vi "main（新）线程二.vi"(8 "停止 2":bool, 11 "线程选择":string(combo)) -> ()   [LabVIEW 2016]
uses:
  <vilib>/Averna/Notify Icon/NotifyIcon.llb/BalloonIcon.ctl
  <vilib>/Utility/miscctls.llb/LVPointTypeDef.ctl
  <vilib>/Utility/config.llb/Read Key (String).vi
  <vilib>/Utility/config.llb/Read Key (I32).vi
  <vilib>/Utility/config.llb/Write Key (String).vi
  <vilib>/Utility/config.llb/Write Key (U32).vi
  <vilib>/Averna/Notify Icon/NotifyIcon.llb/GetSelectedItemEvent.vi
  <vilib>/Averna/Notify Icon/NotifyIcon.llb/SetVisible.vi
  <vilib>/Averna/Notify Icon/NotifyIcon.llb/SetMenuDefaultItem.vi
  <vilib>/Averna/Notify Icon/NotifyIcon.llb/SetTipText.vi
  <vilib>/Averna/Notify Icon/NotifyIcon.llb/NotifyIcon.lvclass
  <vilib>/Utility/config.llb/NI_LVConfig.lvlib
  data/FreeMem.dll
  <vilib>/ptbypt/NI_PtbyPt.lvlib
panel:
  in  "系统编码选择框":string(combo)="地表水质量监测"
  out "主队列输出":refnum<queue>
  out "软件版本":string
  out "数据接收中断 2":bool=TRUE
  out "掉线指示":bool
  out "数据上传":bool
  out "通信状态":bool
  in  "TCP掉线时间节点":string
  out "TCP服务端掉线计数":i32
  out "元素":string
  out "步骤":T1(ring)
  out "1st Error to Convert":i32(ring)=56 items=["无错误", "参数错误", "内存已满", "超出区域", "文件结束", "文件已打开", "一般文件IO错误", "未找到文件", "文件权限错误", "磁盘已满", "路径副本", "打开过多文件", "未启用", "未找到资源文件", "无法添加资源", "未找到资源", "未找到图像", "图像内存错误", "画笔不存在", "配置错误类型", "配置未找到解析段", "配置解析错误", "配置内存错误", "错误外部代码格式", "错误外部代码偏移量", "外部代码不存在", "空窗口", "销毁窗口错误", "空菜单", "打印已中止", "错误打印记录", "打印驱动程序错误", "打印时窗口错误", "打印时内存错误", "打印对话框错误", "一般打印错误", "无效设备引用句柄", "设备未找到", "设备参数错误", "设备单位错误", "无法打开设备", "设备调用已中止", "一般错误", "用户已取消", "对象ID过低", "对象ID过高", "对象不在堆中", "未知的堆", "错误DefProc ID", "DefProc不在表格中", "范围外信息", "空方法", "未知信息", "不支持管理器调用", "错误地址", "连接过程中", "连接超时", "连接过程中", "不支持网络属性", "网络错误", "正在使用的地址", "系统缺少内存", "连接已中止", "连接已拒绝", "连接未建立", "连接已建立", "连接已关闭", "初始化错误（交互应用程序管理器）", "错误事件发生", "等待无约束事件发生处理程序", "事件发生队列溢出", "错误路径", "未发出信号量", "未识别类型（交互应用程序管理器）"]
  out "重发数据":bool
  in  "确定":bool
  out "配置信息":T2
  in  "返回":bool
  in  "参数配置":bool
  in  "PW1":string
  in  "MN1":string
  in  "PORT1":string
  in  "IP1":string
  in  "站点设备1":string
  in  "站点名称1":string
  in  "站点设备":string(combo)="古田污水厂5号"
  in  "站点名称":string(combo)="古田"
  in  "port":string(combo)="1000"
  in  "IP":string(combo)="127.0.0.1"
  in  "PW":string
  in  "MN":string
  out "设置超时时间/min":i32=1
  in  "实时数据发送时间间隔/min":u32=10
  in  "配置模式":u16(ring) items=["现有参数", "自主输入"]
  out "连接的字符串":string
  out "参数":string
  out "data":string[][](table)
  out "数据发送重叠":bool
  out "数据接收中断":bool=TRUE
  out "数据正在发送":bool=TRUE
  out "QN":string
  out "时间QN":string
  out "系统编码ST":string
  out "命令编码CN":string
  out "密码PW":string
  out "设备编码MN":string
  out "拆分包及应答Flag":string
  out "数据":string
  in  "实时数据参数选择框":T3={"水样测量数据"=TRUE, "零点核查数据"=TRUE, "跨度核查数据"=TRUE, "加标回收数据"=TRUE, "平行样数据"=FALSE}
  out "运行时间次数":i32
  out "数据输出":string
  out "try":dbl
  in  "table元素":string
  out "读取报文显示":string
  out "发送报文显示":string
  out "数组":string[](array[string])
  out "数组 2":string[](array[string])
  out "空闲时间":dbl
  out "心跳包":bool
  out "时间标识":timestamp format="%<%Y/%m/%d %H:%M:%S>T"
  in  "连接ID":refnum<k5>
  out "错误输出":errorcluster
  out "主动上传数据次数":i32
  out "error out":errorcluster
  # "192.168.165.122"
  # "3300"
  # "已经实现的功能：发送实时数据、读取小时数据、反控指令、读取核查数据"
  # "数据发送间隔时间必须要小于数采仪出数据的时间间隔"
  # "读取发送的参数要可选择，包括：参数名、因子编码"
  # "参数配置"
  # "站点名称"
  # "站点设备"
  # "IP"
  # "PORT"
  # "MN"
  # "PW"
  # "读取的参数区"
  # "水样测量数据"
  # "零点核查数据"
  # "跨度核查数据"
  # "加标回收数据"
  # "平行样数据"
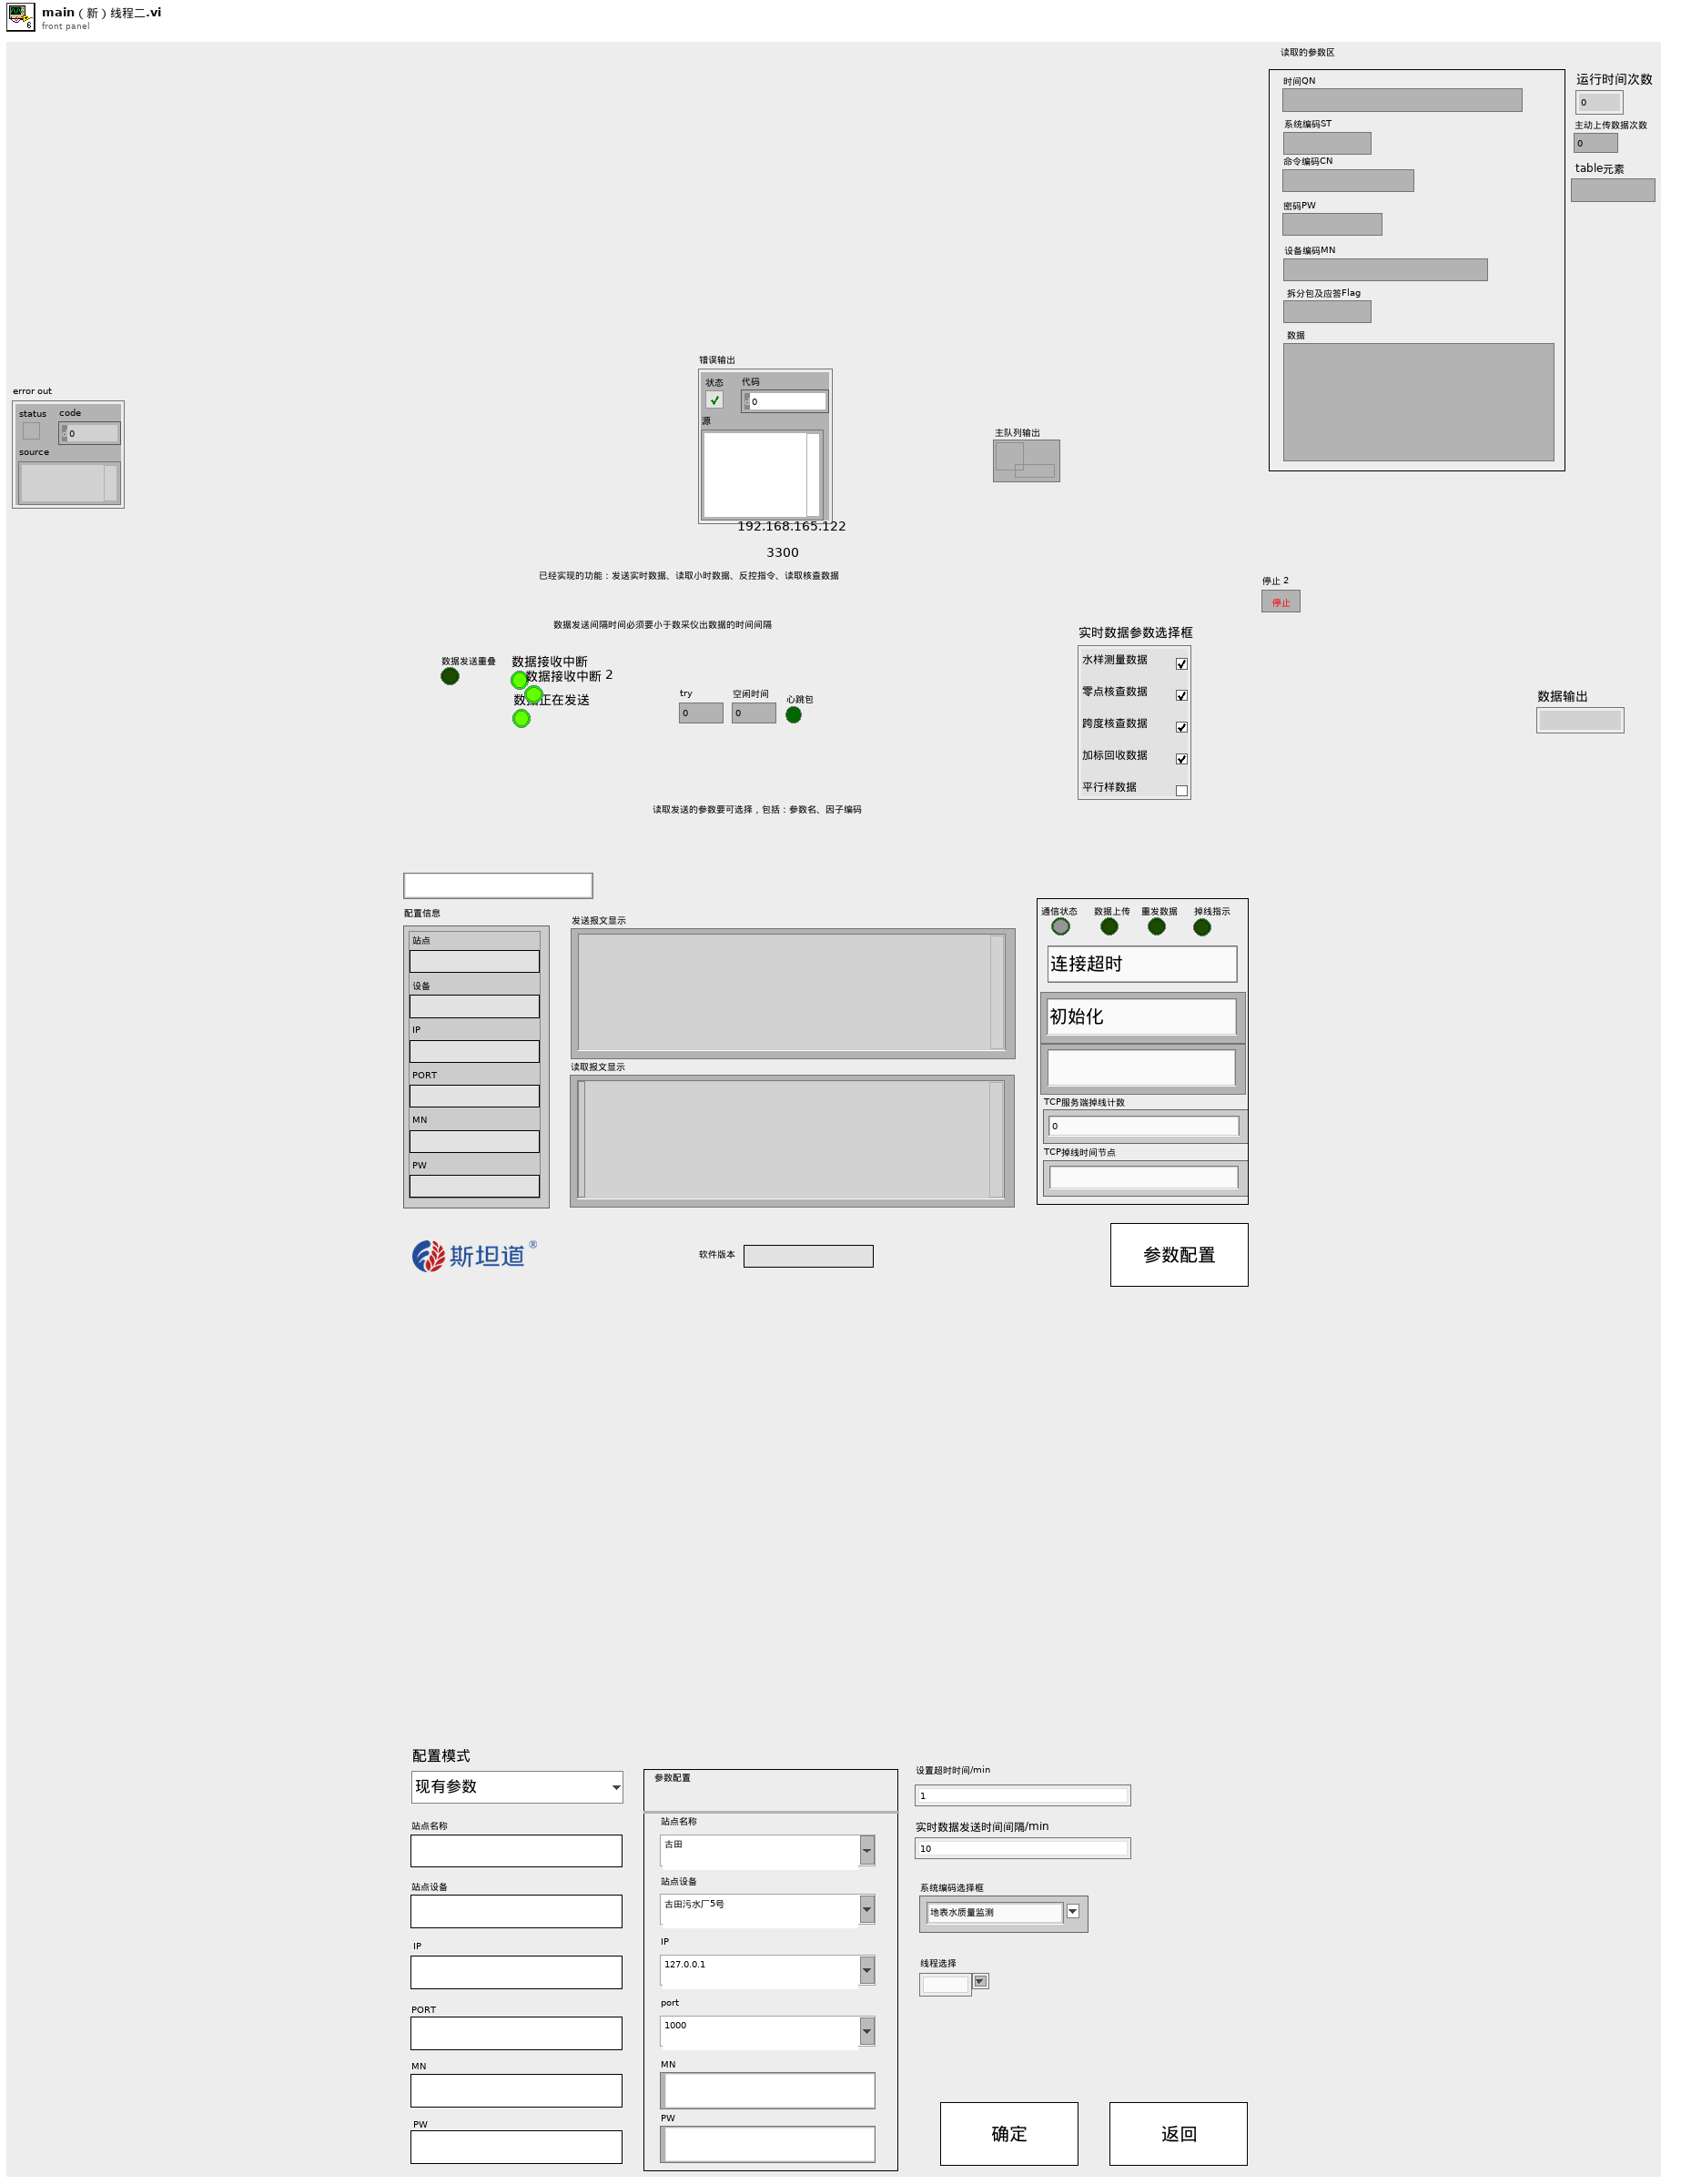
[diagram p1: front panel]
types:
  T1 = enum16{"初始化", "打开连接", "表格比对", "发送数据", "读取数据", "数据处理"}
  T2 = cluster{"站点":string, "设备":string, "IP":string, "PORT":string, "MN":string, "PW":string}
  T3 = cluster{"水样测量数据":bool, "零点核查数据":bool, "跨度核查数据":bool, "加标回收数据":bool, "平行样数据":bool}
  T4 = enum32{"Bad", "Idle", "Run top level", "Running"}
  T5 = typedef "LVPointTypeDef.ctl" = cluster{"Horizontal":i16, "Vertical":i16}
  T6 = typedef "NI_LVConfig.lvlib/Config Data RefNum.ctl" = refnum<k1>
  T7 = enum32{"invalid app kind", "Development System", "Run Time System", "Student Edition", "Embedded LabVIEW", "Evaluation", "Custom"}
  T8 = enum32{"Invalid", "Standard", "Closed", "Hidden", "Minimized", "Maximized"}
  T9 = enum16{"水样测试", "小时数据", "日志信息", "报警信息", "零点核查", "标样核查", "平行样", "加标回收"}
  T10 = enum16{"Standard", "Buffered", "CRLF", "Immediate"}
  T11 = cluster{"高锰酸盐":string, "氨氮":string, "总磷":string, "总氮":string, "数采仪":string, "高锰酸盐":bool, "氨氮":bool, "总磷":bool, "总氮":bool, "数采仪":bool}
  T12 = typedef "NotifyIcon.lvlib/NotifyIcon.lvclass/BalloonIcon.ctl" = enum32{"None", "Information", "Warning", "Error"}
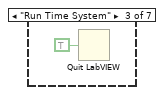
[diagram p3: hidden frame]
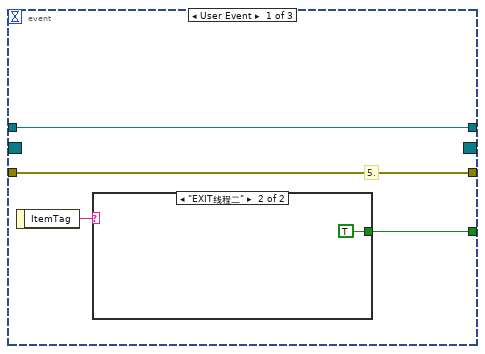
[diagram p9: hidden frame]
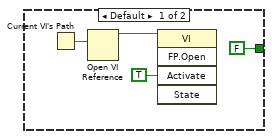
[diagram p10: hidden frame]
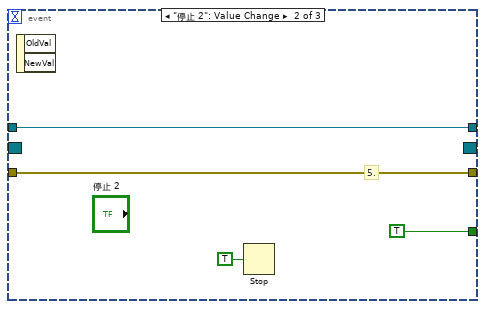
[diagram p11: hidden frame]
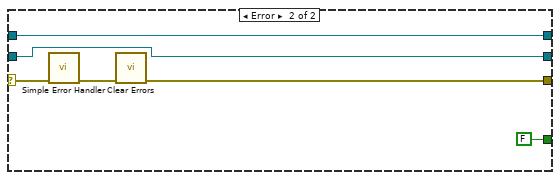
[diagram p12: hidden frame]
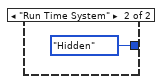
[diagram p13: hidden frame]
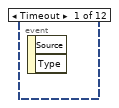
[diagram p15: hidden frame]
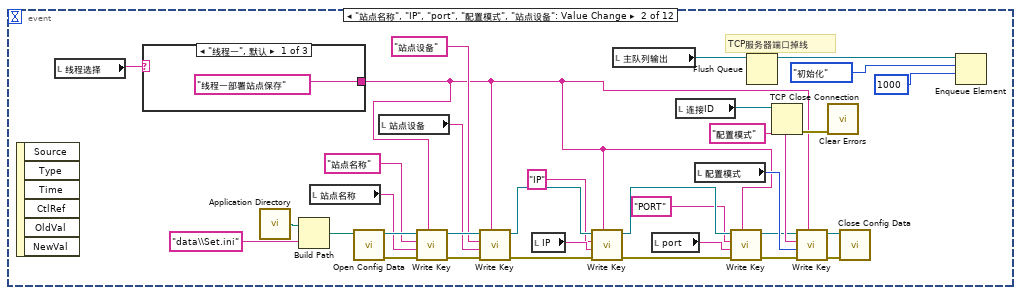
[diagram p16: hidden frame]
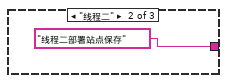
[diagram p17: hidden frame]
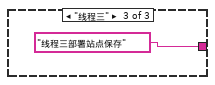
[diagram p18: hidden frame]
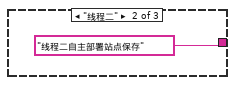
[diagram p19: hidden frame]
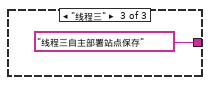
[diagram p20: hidden frame]
diagram:
  w22 = string[] ["OPEN线程二", "APP_SEPARATOR", "EXIT线程二"]
  (unwired) 0 items=["无错误", "参数错误", "内存已满", "超出区域", "文件结束", "文件已打开", "一般文件IO错误", "未找到文件", "文件权限错误", "磁盘已满", "路径副本", "打开过多文件", "未启用", "未找到资源文件", "无法添加资源", "未找到资源", "未找到图像", "图像内存错误", "画笔不存在", "配置错误类型", "配置未找到解析段", "配置解析错误", "配置内存错误", "错误外部代码格式", "错误外部代码偏移量", "外部代码不存在", "空窗口", "销毁窗口错误", "空菜单", "打印已中止", "错误打印记录", "打印驱动程序错误", "打印时窗口错误", "打印时内存错误", "打印对话框错误", "一般打印错误", "无效设备引用句柄", "设备未找到", "设备参数错误", "设备单位错误", "无法打开设备", "设备调用已中止", "一般错误", "用户已取消", "对象ID过低", "对象ID过高", "对象不在堆中", "未知的堆", "错误DefProc ID", "DefProc不在表格中", "范围外信息", "空方法", "未知信息", "不支持管理器调用", "错误地址", "连接过程中", "连接超时", "连接过程中", "不支持网络属性", "网络错误", "正在使用的地址", "系统缺少内存", "连接已中止", "连接已拒绝", "连接未建立", "连接已建立", "连接已关闭", "初始化错误（交互应用程序管理器）", "错误事件发生", "等待无约束事件发生处理程序", "事件发生队列溢出", "错误路径", "未发出信号量", "未识别类型（交互应用程序管理器）"] ("1st Error to Convert")
  # "6."
  # "3."
  # "1."
  # "目前时间太短，如果掉线了，数据存不了临时表格"
  # "3.表格中数据较多的情况下，数据补发送需要分批发送"
  # "1.发送数据过程中突然掉线（如果是查询之后的服务端掉线，不作处理；如果是整点主动上传时掉线，标记数据接收中断，然后数据存入表格）\n2.在查询过程中到了整点要发数据怎么处理（判定查询数据发送完全再进行出列队读取数据）\n3.一般情况掉线，数据存储入临时表格，上线了重发"
  # "判定当数据没有传送完毕并掉线，将数据存储入临时表格"
  # "获取需要发送的数据表"
  n1 = Obtain Queue(name (unnamed)="数据发送" ("名称（未命名）"), element data type="") -> (queue out=w34:refnum<queue>, error out=w33:errorcluster)  [unwired: 3 in, 1 out]
  n2 = Obtain Queue(name (unnamed)="实时数据参数选择" ("名称（未命名）"), element data type="") -> (queue out=w35:refnum<queue>, error out=w32:errorcluster)  [unwired: 3 in, 1 out]
  n3 = while "While循环" {
    tunnel: w34 -> [w66]
    tunnel: w35 -> [w71]
    tunnel: w33 -> [w70]
    tunnel: w32 -> [w69]
    i -> [w72]
    stop <- FALSE stop-if-true
    # "判定数据发送时要发送实时数据"
    # "所有的主动上传数据都是有数据才会上传"
    n4 = Get Queue Status(queue=w66) -> (# elements in queue=w57:i32)  [unwired: 2 in, 7 out]
    n5 = local read "数据正在发送"() -> (w64:bool)
    n6 = global read "全局 实时数据参数.vi" "连接的字符串"() -> (→"连接的字符串":string)
    n7 = global read "全局 实时数据参数.vi" "data"() -> (→"data":string[][])
    n8 = Not Equal To 0?(x=w57) -> (x != 0?=w65:bool)
    n9 = global read "全局 实时数据参数.vi" "参数"() -> (→"参数":string)
    n10 = And(x=w65, y=w64) -> (x .and. y?=w62:bool)
    "数据发送重叠" <- w62
    n11 = call <vilib>:"Boolean Crossing PtByPt.vi"("direction"=enum16{"either", "false-true", "true-false"}."false-true", "input"=w62) -> ("crossing"=w63:bool)  [unwired: 1 in]
    n12 = case shown="真" w63 {
      frame False {
      }
      frame True {
        n13 = Get Date/Time In Seconds() -> (seconds since 1Jan1904=w75:timestamp)
        n14 = Format Date/Time String(time format string (%c)="%Y%m%d%H%M%S%3u" ("时间格式字符串(%c)"), seconds (now)=w75) -> (date/time string=w79:string)  [unwired: 1 in]
        n15 = Search and Replace String(input string=w79, search string="." ("搜索字符串")) -> (result string=w78:string)  [unwired: 6 in, 3 out]
        n16 = call "格式时间字符串.vi"("字符串"=w78) -> ("连接的字符串"=w74:string)  [unwired: 10 in]
        n17 = global write "全局 数据发送重叠.vi" "数据发送重叠开始时间戳"(w74) -> ()
      }
    }
    n18 = Equal To 0?(x=w57) -> (x = 0?=w56:bool)
    n19 = Not(x=w56) -> (.not. x?=w55:bool)
    n20 = Wait (ms)(milliseconds to wait=u32 1000 ("等待时间（毫秒）")) -> ()  [unwired: 1 out]
    n21 = Not(x=w64) -> (.not. x?=w68:bool)
    n22 = local write "数据上传"(w55) -> ()
    n23 = global write "全局 数据发送重叠.vi" "数据发送重叠"(w62) -> ()
    n24 = case shown="真" w68 {
      tunnel: w66 -> [_ w84]
      tunnel: w71 -> [_ w83]
      tunnel: w70 -> [_ w82]
      tunnel: w69 -> [_ w81]
      frame False {
      }
      frame True {
        n25 = Dequeue Element(queue=w84, error in (no error)=w82) -> (element=w80:string)  [unwired: 1 in, 3 out]
        n26 = case shown="\"小时数据\"" w80 {
          tunnel: w83 -> [_ w86 _ _ _]
          tunnel: w81 -> [_ w85 _ _ _]
          frame "假", Default {
          }
          frame "send" {
            # "间隔时间上传"
            n27 = while {
              tunnel: w86 -> [w90]
              tunnel: w85 -> [w87]
              stop <- w91 stop-if-true
              n28 = Dequeue Element(queue=w90, error in (no error)=w87) -> (queue out=w89:refnum<queue>, element=w92:string)  [unwired: 1 in, 2 out]
              n29 = case shown="\"水样测量数据\"" w92 {
                tunnel: [_ _ _ _ _ w234] -> w91
                tunnel: w89 -> [_ _ _ _ _ w237]
                frame "水样测量数据" {
                  n30 = flat-sequence {
                    frame #0 {
                      n31 = global write "全局 小时数据发送次数.vi" "小时数据发送次数"(0 ("小时数据发送次数")) -> ()
                      n32 = global write "全局 实时数据参数.vi" "实时数据参数"("水样测试") -> ()
                      n33 = global write "全局1.vi" "枚举"(enum16{"返回请求应答", "上传数据", "返回执行结果"}."上传数据" ("枚举")) -> ()
                    }
                    frame #1 {
                      n34 = call "从数据库获取数据通用可配置(子VI).vi"("table输入"="实时数据" ("新元素/子数组"), "列队名（唯一）"="a") -> ()  [unwired: 8 in, 2 out]
                    }
                    frame #2 {
                      n35 = call "实时小时数据处理整合 (子VI).vi"("枚举"=enum16{"实时数据排序", "小时数据排序"}."实时数据排序") -> ("已排序的数组"=w99:string[])  [unwired: 10 in]
                      n36 = Array Size(array=w99) -> (size(s)=w100:i32)
                      n37 = global write "全局 数据数组大小.vi" "数据数组大小"(w100) -> ()
                    }
                    frame #3 {
                      n38 = while {
                        stop <- w105 stop-if-true
                        n39 = property on="TCP服务端掉线计数" class="DigNum (严格)"() -> ("Value"=w108:i32)  [unwired: 2 in, 2 out]
                        n40 = Greater Or Equal?(x=w108, y=1) -> (x >= y?=w107:bool)
                        n41 = case shown="假" w107 {
                          frame False {
                            n42 = global read "全局 数据数组大小.vi" "数据数组大小"() -> (w110:i32)
                            n43 = Greater Than 0?(x=w110) -> (x > 0?=w111:bool)
                            n44 = case shown="真" w111 {
                              frame False {
                              }
                              frame True {
                                n45 = local read "MN"() -> (w117:string)
                                n46 = local read "PW"() -> (w116:string)
                                n47 = call "数据编码.vi"("table输入"="实时数据" ("新元素/子数组"), "MN"=w117, "PW"=w116) -> ("通讯包字符串"=w115:string)  [unwired: 11 in, 1 out]
                                n48 = local write "发送报文显示"(w115) -> ()
                                n49 = TCP Write(connection ID="连接ID", data in=w115) -> (error out=→"错误输出":errorcluster)  [unwired: 2 in, 2 out]
                                n50 = Build Array(w115) -> (w114:string[])
                                n51 = call "发送数据记录到文档(子VI).vi"("数组"=w114) -> ()  [unwired: 9 in, 1 out]
                                "数据上传" <- TRUE ("主动数据上传")
                              }
                            }
                          }
                          frame True {
                          }
                        }
                        n52 = Wait (ms)(milliseconds to wait=u32 500 ("等待时间（毫秒）")) -> ()  [unwired: 1 out]
                        n53 = global read "全局 数据数组大小.vi" "数据数组大小"() -> (w102:i32)
                        n54 = global read "全局 小时数据发送次数.vi" "小时数据发送次数"() -> (w106:i32)
                        n55 = Decrement(x=w102) -> (x-1=w101:i32)
                        n56 = Greater Or Equal?(x=w106, y=w101) -> (x >= y?=w104:bool)
                        n57 = Compound Arithmetic op=OR ("复合运算")(w104) -> (w105:bool)
                      }
                    }
                  }
                }
                frame "零点核查数据" {
                  n58 = flat-sequence {
                    frame #0 {
                      n59 = global write "全局 小时数据发送次数.vi" "小时数据发送次数"(0 ("小时数据发送次数")) -> ()
                      n60 = global write "全局 实时数据参数.vi" "实时数据参数"("空白测试") -> ()
                      n61 = global write "全局1.vi" "枚举"(enum16{"返回请求应答", "上传数据", "返回执行结果"}."上传数据" ("枚举")) -> ()
                    }
                    frame #1 {
                      n62 = call "从数据库获取数据通用可配置(子VI).vi"("table输入"="实时数据" ("新元素/子数组"), "列队名（唯一）"="b") -> ()  [unwired: 8 in, 2 out]
                    }
                    frame #2 {
                      n63 = call "数据处理整合 (子VI).vi"("枚举"=enum16{"实时数据排序", "小时数据排序"}."实时数据排序") -> ("已排序的数组"=w127:string[])  [unwired: 10 in]
                      n64 = Array Size(array=w127) -> (size(s)=w126:i32)
                      n65 = global write "全局 数据数组大小.vi" "数据数组大小"(w126) -> ()
                    }
                    frame #3 {
                      n66 = while {
                        stop <- w130 stop-if-true
                        n67 = property on="TCP服务端掉线计数" class="DigNum (严格)"() -> ("Value"=w135:i32)  [unwired: 2 in, 2 out]
                        n68 = Greater Or Equal?(x=w135, y=1) -> (x >= y?=w134:bool)
                        n69 = case shown="假" w134 {
                          frame False {
                            n70 = global read "全局 数据数组大小.vi" "数据数组大小"() -> (w138:i32)
                            n71 = Greater Than 0?(x=w138) -> (x > 0?=w137:bool)
                            n72 = case shown="真" w137 {
                              frame False {
                              }
                              frame True {
                                n73 = local read "MN"() -> (w145:string)
                                n74 = local read "PW"() -> (w144:string)
                                n75 = local write "数据上传"(TRUE ("数据上传")) -> ()
                                n76 = local read "连接ID"() -> (w143:refnum<k5>)
                                n77 = call "数据编码.vi"("table输入"="实时数据" ("新元素/子数组"), "MN"=w145, "PW"=w144) -> ("通讯包字符串"=w141:string)  [unwired: 11 in, 1 out]
                                n78 = local write "发送报文显示"(w141) -> ()
                                n79 = TCP Write(connection ID=w143, data in=w141) -> (error out=w142:errorcluster)  [unwired: 2 in, 2 out]
                                n80 = Build Array(w141) -> (w140:string[])
                                n81 = call "发送数据记录到文档(子VI).vi"("数组"=w140) -> ()  [unwired: 9 in, 1 out]
                                n82 = local write "错误输出"(w142) -> ()
                              }
                            }
                          }
                          frame True {
                          }
                        }
                        n83 = Wait (ms)(milliseconds to wait=u32 500 ("等待时间（毫秒）")) -> ()  [unwired: 1 out]
                        n84 = global read "全局 数据数组大小.vi" "数据数组大小"() -> (w133:i32)
                        n85 = global read "全局 小时数据发送次数.vi" "小时数据发送次数"() -> (w132:i32)
                        n86 = Decrement(x=w133) -> (x-1=w129:i32)
                        n87 = Greater Or Equal?(x=w132, y=w129) -> (x >= y?=w131:bool)
                        n88 = Compound Arithmetic op=OR ("复合运算")(w131) -> (w130:bool)
                      }
                    }
                  }
                }
                frame "跨度核查数据" {
                  n89 = flat-sequence {
                    frame #0 {
                      n90 = global write "全局 小时数据发送次数.vi" "小时数据发送次数"(0 ("小时数据发送次数")) -> ()
                      n91 = global write "全局 实时数据参数.vi" "实时数据参数"("跨度核查") -> ()
                      n92 = global write "全局1.vi" "枚举"(enum16{"返回请求应答", "上传数据", "返回执行结果"}."上传数据" ("枚举")) -> ()
                    }
                    frame #1 {
                      n93 = call "从数据库获取数据通用可配置(子VI).vi"("table输入"="实时数据" ("新元素/子数组"), "列队名（唯一）"="c") -> ()  [unwired: 8 in, 2 out]
                    }
                    frame #2 {
                      n94 = call "数据处理整合 (子VI).vi"("枚举"=enum16{"实时数据排序", "小时数据排序"}."实时数据排序") -> ("已排序的数组"=w154:string[])  [unwired: 10 in]
                      n95 = Array Size(array=w154) -> (size(s)=w153:i32)
                      n96 = global write "全局 数据数组大小.vi" "数据数组大小"(w153) -> ()
                    }
                    frame #3 {
                      n97 = while {
                        stop <- w157 stop-if-true
                        n98 = property on="TCP服务端掉线计数" class="DigNum (严格)"() -> ("Value"=w162:i32)  [unwired: 2 in, 2 out]
                        n99 = property on="TCP服务端掉线计数" class="DigNum (严格)" props=["Value"]() -> ()  [unwired: 2 in, 3 out]
                        n100 = Greater Or Equal?(x=w162, y=1) -> (x >= y?=w161:bool)
                        n101 = case shown="假" w161 {
                          frame False {
                            n102 = global read "全局 数据数组大小.vi" "数据数组大小"() -> (w165:i32)
                            n103 = Greater Than 0?(x=w165) -> (x > 0?=w164:bool)
                            n104 = case shown="真" w164 {
                              frame False {
                              }
                              frame True {
                                n105 = local read "QN"() -> (w169:string)
                                n106 = local read "MN"() -> (w173:string)
                                n107 = local read "PW"() -> (w172:string)
                                n108 = local read "连接ID"() -> (w171:refnum<k5>)
                                n109 = local write "数据上传"(TRUE ("数据上传")) -> ()
                                n110 = call "数据编码.vi"("table输入"="实时数据" ("新元素/子数组"), "QN"=w169, "MN"=w173, "PW"=w172) -> ("通讯包字符串"=w168:string)  [unwired: 10 in, 1 out]
                                n111 = local write "发送报文显示"(w168) -> ()
                                n112 = TCP Write(connection ID=w171, data in=w168) -> (error out=w170:errorcluster)  [unwired: 2 in, 2 out]
                                n113 = Build Array(w168) -> (w167:string[])
                                n114 = local write "错误输出"(w170) -> ()
                                n115 = call "发送数据记录到文档(子VI).vi"("数组"=w167) -> ()  [unwired: 9 in, 1 out]
                              }
                            }
                          }
                          frame True {
                          }
                        }
                        n116 = Wait (ms)(milliseconds to wait=u32 500 ("等待时间（毫秒）")) -> ()  [unwired: 1 out]
                        n117 = global read "全局 数据数组大小.vi" "数据数组大小"() -> (w160:i32)
                        n118 = global read "全局 小时数据发送次数.vi" "小时数据发送次数"() -> (w159:i32)
                        n119 = Decrement(x=w160) -> (x-1=w156:i32)
                        n120 = Greater Or Equal?(x=w159, y=w156) -> (x >= y?=w158:bool)
                        n121 = Compound Arithmetic op=OR ("复合运算")(w158) -> (w157:bool)
                      }
                    }
                  }
                }
                frame "加标回收数据" {
                  n122 = flat-sequence {
                    frame #0 {
                      n123 = global write "全局 小时数据发送次数.vi" "小时数据发送次数"(0 ("小时数据发送次数")) -> ()
                      n124 = global write "全局 实时数据参数.vi" "实时数据参数"("加标回收测试") -> ()
                      n125 = global write "全局1.vi" "枚举"(enum16{"返回请求应答", "上传数据", "返回执行结果"}."上传数据" ("枚举")) -> ()
                    }
                    frame #1 {
                      n126 = call "从数据库获取数据通用可配置(子VI).vi"("table输入"="加标回收" ("新元素/子数组"), "列队名（唯一）"="d") -> ()  [unwired: 8 in, 2 out]
                    }
                    frame #2 {
                      n127 = call "加标回收数据处理整合 (子VI).vi"("枚举"=enum16{"实时数据排序", "小时数据排序"}."实时数据排序") -> ("已排序的数组"=w181:string[])  [unwired: 10 in]
                      n128 = Array Size(array=w181) -> (size(s)=w182:i32)
                      n129 = global write "全局 数据数组大小.vi" "数据数组大小"(w182) -> ()
                    }
                    frame #3 {
                      n130 = while {
                        stop <- w185 stop-if-true
                        n131 = property on="TCP服务端掉线计数" class="DigNum (严格)"() -> ("Value"=w191:i32)  [unwired: 2 in, 2 out]
                        n132 = Greater Or Equal?(x=w191, y=1) -> (x >= y?=w189:bool)
                        n133 = case shown="假" w189 {
                          frame False {
                            n134 = global read "全局 数据数组大小.vi" "数据数组大小"() -> (w193:i32)
                            n135 = Greater Than 0?(x=w193) -> (x > 0?=w192:bool)
                            n136 = case shown="真" w192 {
                              frame False {
                              }
                              frame True {
                                n137 = local read "MN"() -> (w203:string)
                                n138 = Get Date/Time In Seconds() -> (seconds since 1Jan1904=w197:timestamp)
                                n139 = local read "PW"() -> (w204:string)
                                n140 = local read "连接ID"() -> (w205:refnum<k5>)
                                n141 = call "数据编码.vi"("table输入"="实时数据" ("新元素/子数组"), "MN"=w203, "PW"=w204) -> ("通讯包字符串"=w201:string)  [unwired: 11 in, 1 out]
                                n142 = Format Date/Time String(time format string (%c)="%Y/%m/%d %H:%M:%S" ("格式字符串"), seconds (now)=w197) -> (date/time string=w196:string)  [unwired: 1 in]
                                n143 = local write "发送报文显示"(w201) -> ()
                                n144 = TCP Write(connection ID=w205, data in=w201) -> (error out=w206:errorcluster)  [unwired: 2 in, 2 out]
                                n145 = Search and Replace String(input string=w196, search string="." ("搜索字符串")) -> (result string=w198:string)  [unwired: 6 in, 3 out]
                                n146 = Build Array(w201) -> (w200:string[])
                                n147 = global write "全局 时间2.vi" "加标回收索引起始时间"(w198) -> ()
                                n148 = local write "数据上传"(TRUE ("数据上传")) -> ()
                                n149 = local write "错误输出"(w206) -> ()
                                n150 = call "发送数据记录到文档(子VI).vi"("数组"=w200) -> ()  [unwired: 9 in, 1 out]
                              }
                            }
                          }
                          frame True {
                          }
                        }
                        n151 = Wait (ms)(milliseconds to wait=u32 500 ("等待时间（毫秒）")) -> ()  [unwired: 1 out]
                        n152 = global read "全局 数据数组大小.vi" "数据数组大小"() -> (w188:i32)
                        n153 = global read "全局 小时数据发送次数.vi" "小时数据发送次数"() -> (w187:i32)
                        n154 = Decrement(x=w188) -> (x-1=w184:i32)
                        n155 = Greater Or Equal?(x=w187, y=w184) -> (x >= y?=w186:bool)
                        n156 = Compound Arithmetic op=OR ("复合运算")(w186) -> (w185:bool)
                      }
                    }
                  }
                }
                frame "平行样数据" {
                  n157 = flat-sequence {
                    frame #0 {
                      n158 = global write "全局 小时数据发送次数.vi" "小时数据发送次数"(0 ("小时数据发送次数")) -> ()
                      n159 = global write "全局 实时数据参数.vi" "实时数据参数"("平行样测试") -> ()
                      n160 = global write "全局1.vi" "枚举"(enum16{"返回请求应答", "上传数据", "返回执行结果"}."上传数据" ("枚举")) -> ()
                    }
                    frame #1 {
                      n161 = call "从数据库获取数据通用可配置(子VI).vi"("table输入"="实时数据" ("新元素/子数组"), "列队名（唯一）"="e") -> ()  [unwired: 8 in, 2 out]
                    }
                    frame #2 {
                      n162 = call "数据处理整合 (子VI).vi"("枚举"=enum16{"实时数据排序", "小时数据排序"}."实时数据排序") -> ("已排序的数组"=w214:string[])  [unwired: 10 in]
                      n163 = Array Size(array=w214) -> (size(s)=w213:i32)
                      n164 = global write "全局 数据数组大小.vi" "数据数组大小"(w213) -> ()
                    }
                    frame #3 {
                      n165 = while {
                        stop <- w217 stop-if-true
                        n166 = property on="TCP服务端掉线计数" class="DigNum (严格)"() -> ("Value"=w223:i32)  [unwired: 2 in, 2 out]
                        n167 = property on="TCP服务端掉线计数" class="DigNum (严格)" props=["Value"]() -> ()  [unwired: 2 in, 3 out]
                        n168 = Greater Or Equal?(x=w223, y=1) -> (x >= y?=w221:bool)
                        n169 = case shown="假" w221 {
                          frame False {
                            n170 = global read "全局 数据数组大小.vi" "数据数组大小"() -> (w225:i32)
                            n171 = Greater Than 0?(x=w225) -> (x > 0?=w224:bool)
                            n172 = case shown="真" w224 {
                              frame False {
                              }
                              frame True {
                                n173 = local read "MN"() -> (w230:string)
                                n174 = local read "PW"() -> (w231:string)
                                n175 = local read "连接ID"() -> (w232:refnum<k5>)
                                n176 = local write "数据上传"(TRUE ("数据上传")) -> ()
                                n177 = call "数据编码.vi"("table输入"="实时数据" ("新元素/子数组"), "MN"=w230, "PW"=w231) -> ("通讯包字符串"=w228:string)  [unwired: 11 in, 1 out]
                                n178 = local write "发送报文显示"(w228) -> ()
                                n179 = TCP Write(connection ID=w232, data in=w228) -> (error out=w233:errorcluster)  [unwired: 2 in, 2 out]
                                n180 = Build Array(w228) -> (w227:string[])
                                n181 = call "发送数据记录到文档(子VI).vi"("数组"=w227) -> ()  [unwired: 9 in, 1 out]
                                n182 = local write "错误输出"(w233) -> ()
                              }
                            }
                          }
                          frame True {
                          }
                        }
                        n183 = Wait (ms)(milliseconds to wait=u32 500 ("等待时间（毫秒）")) -> ()  [unwired: 1 out]
                        n184 = global read "全局 数据数组大小.vi" "数据数组大小"() -> (w220:i32)
                        n185 = global read "全局 小时数据发送次数.vi" "小时数据发送次数"() -> (w219:i32)
                        n186 = Decrement(x=w220) -> (x-1=w216:i32)
                        n187 = Greater Or Equal?(x=w219, y=w216) -> (x >= y?=w218:bool)
                        n188 = Compound Arithmetic op=OR ("复合运算")(w218) -> (w217:bool)
                      }
                    }
                  }
                }
                frame "", Default {
                  n189 = Get Queue Status(queue=w237) -> (# elements in queue=w236:i32)  [unwired: 2 in, 7 out]
                  n190 = Equal To 0?(x=w236) -> (x = 0?=w235:bool)
                  n191 = case shown="真" w235 {
                    tunnel: [_ TRUE] -> w234
                    frame False {
                    }
                    frame True {
                    }
                  }
                }
              }
              n192 = Wait (ms)(milliseconds to wait=u32 3000 ("等待时间（毫秒）")) -> ()  [unwired: 1 out]
            }
          }
          frame "小时数据" {
            # "间隔时间上传"
            n193 = flat-sequence {
              frame #0 {
                # "发送前2小时的数据"
                n194 = global write "全局 小时数据发送次数.vi" "小时数据发送次数"(1 ("小时数据发送次数")) -> ()
                n195 = global write "全局1.vi" "枚举"(enum16{"返回请求应答", "上传数据", "返回执行结果"}."上传数据" ("枚举")) -> ()
              }
              frame #1 {
                n196 = call "从数据库获取数据通用可配置(子VI).vi"("table输入"="小时数据" ("新元素/子数组"), "列队名（唯一）"="XS" ("名称（未命名）")) -> ()  [unwired: 8 in, 2 out]
              }
              frame #2 {
                n197 = property on="TCP服务端掉线计数" class="DigNum (严格)"() -> ("Value"=w244:i32)  [unwired: 2 in, 2 out]
                n198 = Greater Or Equal?(x=w244, y=1) -> (x >= y?=w243:bool)
                n199 = case shown="假" w243 {
                  frame False {
                    # "数据处理整合"
                    n200 = call "实时小时数据处理整合 (子VI).vi"("枚举"=enum16{"实时数据排序", "小时数据排序"}."小时数据排序") -> ("已排序的数组"=w246:string[])  [unwired: 10 in]
                    n201 = Array Size(array=w246) -> (size(s)=w249:i32)
                    n202 = global write "全局 数据数组大小.vi" "数据数组大小"(1 ("数据数组大小")) -> ()
                    n203 = Greater Than 0?(x=w249) -> (x > 0?=w250:bool)
                    n204 = case shown="真" w250 {
                      frame False {
                      }
                      frame True {
                        n205 = local write "数据上传"(TRUE ("数据上传")) -> ()
                        n206 = Get Date/Time In Seconds() -> (seconds since 1Jan1904=w260:timestamp)
                        n207 = Format Date/Time String(time format string (%c)="%Y%m%d%H%M%S%3u" ("时间格式字符串(%c)"), seconds (now)=w260) -> (date/time string=w261:string)  [unwired: 1 in]
                        n208 = local read "连接ID"() -> (w254:refnum<k5>)
                        n209 = local read "MN"() -> (w256:string)
                        n210 = local read "PW"() -> (w257:string)
                        n211 = Search and Replace String(input string=w261, search string="." ("搜索字符串")) -> (result string=w263:string)  [unwired: 6 in, 3 out]
                        n212 = call "数据编码.vi"("table输入"="小时数据" ("新元素/子数组"), "QN"=w263, "MN"=w256, "PW"=w257) -> ("通讯包字符串"=w253:string)  [unwired: 10 in, 1 out]
                        n213 = local write "发送报文显示"(w253) -> ()
                        n214 = TCP Write(connection ID=w254, data in=w253) -> (error out=w258:errorcluster)  [unwired: 2 in, 2 out]
                        n215 = Build Array(w253) -> (w252:string[])
                        n216 = local write "错误输出"(w258) -> ()
                        n217 = call "发送数据记录到文档(子VI).vi"("数组"=w252) -> ()  [unwired: 9 in, 1 out]
                      }
                    }
                  }
                  frame True {
                  }
                }
              }
            }
          }
          frame "操作日志" {
            # "间隔时间上传"
            # "直接1分钟查询 一次,有数据就按数据上传,没数据就不上传,在数据发送那边有做处理"
            n218 = flat-sequence {
              frame #0 {
                # "时间"
                n219 = global read "全局 数据发送重叠.vi" "数据发送重叠开始时间戳"() -> (w265:string)
                n220 = global read "全局 数据发送重叠.vi" "数据发送重叠"() -> (w264:bool)
                n221 = global write "全局 小时数据发送次数.vi" "小时数据发送次数"(0 ("小时数据发送次数")) -> ()
                n222 = global write "全局1.vi" "枚举"(enum16{"返回请求应答", "上传数据", "返回执行结果"}."上传数据" ("枚举")) -> ()
                n223 = call "日志信息主动发送(子VI).vi"("是否正在查询数据"=w264, "查询数据发送时间节点"=w265) -> ()  [unwired: 10 in]
              }
              frame #1 {
                n224 = call "获取操作日志 (子VI).vi"() -> ()  [unwired: 12 in]
              }
              frame #2 {
                n225 = call "数据处理整合 (子VI).vi"("枚举"=enum16{"实时数据排序", "小时数据排序"}."实时数据排序") -> ("已排序的数组"=w270:string[])  [unwired: 10 in]
                n226 = Array Size(array=w270) -> (size(s)=w269:i32)
                n227 = global write "全局 数据数组大小.vi" "数据数组大小"(w269) -> ()
              }
              frame #3 {
                # "判定是否存表"
                n228 = property on="TCP服务端掉线计数" class="DigNum (严格)"() -> ("Value"=w272:i32)  [unwired: 2 in, 2 out]
                n229 = Greater Or Equal?(x=w272, y=1) -> (x >= y?=w271:bool)
                n230 = case shown="假" w271 {
                  frame False {
                    n231 = global read "全局 数据数组大小.vi" "数据数组大小"() -> (w274:i32)
                    n232 = Greater Than 0?(x=w274) -> (x > 0?=w275:bool)
                    n233 = case shown="真" w275 {
                      frame False {
                      }
                      frame True {
                        n234 = global read "全局 小时数据发送次数.vi" "小时数据发送次数"() -> (w278:i32)
                        n235 = local write "数据上传"(TRUE ("数据上传")) -> ()
                        n236 = Get Date/Time In Seconds() -> (seconds since 1Jan1904=w284:timestamp)
                        n237 = Increment(x=w278) -> (x+1=w277:i32)
                        n238 = Format Date/Time String(time format string (%c)="%Y%m%d%H%M%S%3u" ("时间格式字符串(%c)"), seconds (now)=w284) -> (date/time string=w283:string)  [unwired: 1 in]
                        n239 = global write "全局 小时数据发送次数.vi" "小时数据发送次数"(w277) -> ()
                        n240 = Search and Replace String(input string=w283, search string="." ("搜索字符串")) -> (result string=w281:string)  [unwired: 6 in, 3 out]
                        n241 = local read "MN"() -> (w288:string)
                        n242 = local read "连接ID"() -> (w290:refnum<k5>)
                        n243 = local read "PW"() -> (w287:string)
                        n244 = call "数据编码.vi"("table输入"="操作日志" ("新元素/子数组"), "QN"=w281, "MN"=w288, "PW"=w287) -> ("通讯包字符串"=w280:string)  [unwired: 10 in, 1 out]
                        n245 = local write "发送报文显示"(w280) -> ()
                        n246 = TCP Write(connection ID=w290, data in=w280) -> (error out=w286:errorcluster)  [unwired: 2 in, 2 out]
                        n247 = Build Array(w280) -> (w279:string[])
                        n248 = local write "错误输出"(w286) -> ()
                        n249 = call "发送数据记录到文档(子VI).vi"("数组"=w279) -> ()  [unwired: 9 in, 1 out]
                      }
                    }
                  }
                  frame True {
                  }
                }
              }
            }
          }
          frame "报警信息" {
            # "间隔时间上传"
            # "直接1分钟查询 一次,有数据就按数据上传,没数据就空的上传,在数据发送那边有做处理"
            n250 = flat-sequence {
              frame #0 {
                # "分钟时间间隔"
                n251 = global read "全局 数据发送重叠.vi" "数据发送重叠开始时间戳"() -> (w292:string)
                n252 = global read "全局 数据发送重叠.vi" "数据发送重叠"() -> (w291:bool)
                n253 = global write "全局 小时数据发送次数.vi" "小时数据发送次数"(0 ("小时数据发送次数")) -> ()
                n254 = global write "全局1.vi" "枚举"(enum16{"返回请求应答", "上传数据", "返回执行结果"}."上传数据" ("枚举")) -> ()
                n255 = call "日志信息主动发送(子VI).vi"("是否正在查询数据"=w291, "查询数据发送时间节点"=w292) -> ()  [unwired: 10 in]
              }
              frame #1 {
                n256 = call "获取报警信息 (子VI).vi"() -> ()  [unwired: 12 in]
              }
              frame #2 {
                n257 = call "数据处理整合 (子VI).vi"("枚举"=enum16{"实时数据排序", "小时数据排序"}."实时数据排序") -> ("已排序的数组"=w297:string[])  [unwired: 10 in]
                n258 = Array Size(array=w297) -> (size(s)=w296:i32)
                n259 = global write "全局 数据数组大小.vi" "数据数组大小"(w296) -> ()
              }
              frame #3 {
                # "判定是否存表"
                n260 = property on="TCP服务端掉线计数" class="DigNum (严格)"() -> ("Value"=w299:i32)  [unwired: 2 in, 2 out]
                n261 = Greater Or Equal?(x=w299, y=1) -> (x >= y?=w298:bool)
                n262 = case shown="假" w298 {
                  frame False {
                    # "判定数据不为空才发"
                    n263 = global read "全局 数据数组大小.vi" "数据数组大小"() -> (w301:i32)
                    n264 = Greater Than 0?(x=w301) -> (x > 0?=w302:bool)
                    n265 = case shown="真" w302 {
                      frame False {
                      }
                      frame True {
                        n266 = global read "全局 小时数据发送次数.vi" "小时数据发送次数"() -> (w305:i32)
                        n267 = local write "数据上传"(TRUE ("数据上传")) -> ()
                        n268 = Get Date/Time In Seconds() -> (seconds since 1Jan1904=w311:timestamp)
                        n269 = Increment(x=w305) -> (x+1=w304:i32)
                        n270 = Format Date/Time String(time format string (%c)="%Y%m%d%H%M%S%3u" ("时间格式字符串(%c)"), seconds (now)=w311) -> (date/time string=w310:string)  [unwired: 1 in]
                        n271 = global write "全局 小时数据发送次数.vi" "小时数据发送次数"(w304) -> ()
                        n272 = Search and Replace String(input string=w310, search string="." ("搜索字符串")) -> (result string=w308:string)  [unwired: 6 in, 3 out]
                        n273 = local read "MN"() -> (w315:string)
                        n274 = local read "连接ID"() -> (w317:refnum<k5>)
                        n275 = local read "PW"() -> (w314:string)
                        n276 = call "数据编码.vi"("table输入"="报警信息" ("新元素/子数组"), "QN"=w308, "MN"=w315, "PW"=w314) -> ("通讯包字符串"=w307:string)  [unwired: 10 in, 1 out]
                        n277 = local write "发送报文显示"(w307) -> ()
                        n278 = TCP Write(connection ID=w317, data in=w307) -> (error out=w313:errorcluster)  [unwired: 2 in, 2 out]
                        n279 = Build Array(w307) -> (w306:string[])
                        n280 = local write "错误输出"(w313) -> ()
                        n281 = call "发送数据记录到文档(子VI).vi"("数组"=w306) -> ()  [unwired: 9 in, 1 out]
                      }
                    }
                  }
                  frame True {
                  }
                }
              }
            }
          }
        }
      }
    }
    "主动上传数据次数" <- w72
  }
  n282 = while {
    tunnel: w34 -> [w323]
    stop <- FALSE stop-if-true
    # "整点发送"
    # "小时数据只针对水样测试的值"
    # "整点发送小时数据"
    n283 = Multiply(x=u32 1, y=u32 60000 ("等待时间（毫秒）")) -> (x*y=w333:u32)
    n284 = Get Date/Time In Seconds() -> (seconds since 1Jan1904=w327:timestamp)
    n285 = Wait (ms)(milliseconds to wait=w333) -> ()  [unwired: 1 out]
    n286 = Format Date/Time String(time format string (%c)="%Y%m%d%H%M%S%3u" ("时间格式字符串(%c)"), seconds (now)=w327) -> (date/time string=w328:string)  [unwired: 1 in]
    n287 = String Subset(string=w328, offset (0)=10 ("偏移量(0)"), length (rest)=2 ("长度（剩余）")) -> (substring=w325:string)
    n288 = Equal?(x=w325, y="00") -> (x = y?=w318:bool)
    n289 = case shown="真" w318 {
      tunnel: w323 -> [_ w335]
      frame False {
      }
      frame True {
        # "获取小时数据时间段"
        n290 = Enqueue Element(queue=w335, element="小时数据" ("元素")) -> ()  [unwired: 2 in, 3 out]
        n291 = call "小时数据主动发送(子VI).vi"() -> ()  [unwired: 12 in]
      }
    }
    n292 = Enqueue Element(queue=w323, element="操作日志" ("元素")) -> (queue out=w321:refnum<queue>, error out=w320:errorcluster)  [unwired: 2 in, 1 out]
    n293 = Enqueue Element(queue=w321, element="报警信息" ("元素"), error in (no error)=w320) -> ()  [unwired: 1 in, 3 out]
  }
  n294 = while {
    tunnel: w34 -> [w344]
    stop <- FALSE stop-if-true
    # "核查和质控数据的定期发送在实时数据周期上传"
    # "指定周期发一次实时小时数据"
    n295 = Enqueue Element(queue=w344, element="send" ("元素")) -> ()  [unwired: 2 in, 3 out]
    n296 = Multiply(x="实时数据发送时间间隔/min", y=u32 60000 ("等待时间（毫秒）")) -> (x*y=w342:u32)
    n297 = First Call?() -> (First Call?: T/F=w337:bool)
    n298 = Wait (ms)(milliseconds to wait=w342) -> ()  [unwired: 1 out]
    n299 = case shown="真" w337 {
      frame False {
      }
      frame True {
        n300 = global write "全局 时间2.vi" "加标回收索引起始时间"("1904/01/01 00:00:00") -> ()
      }
    }
    n301 = call "实时数据参数入列队.vi"("发送实时数据选择框"="实时数据参数选择框") -> ("错误输出"=w339:errorcluster)  [unwired: 10 in]
    n302 = call <vilib>:"Clear Errors.vi"("error in (no error)"=w339) -> ()  [unwired: 5 in, 2 out]
  }
  n303 = disable-structure shown="禁用" {
    frame Disabled {
      n304 = vi-ref "Modbus Master.vi"() -> (w347:refnum<vi>)
      n305 = property class="VI"(reference=w347) -> (reference out=w349:refnum<vi>, "Exec.State"=w348:T4)  [unwired: 1 in, 1 out]
      n306 = case shown="\"Idle\"" w348 {
        tunnel: w349 -> [_ w352]
        frame "Bad", Default {
        }
        frame "Idle" {
          n307 = invoke class="VI" method="Run VI"(reference=w352, "Wait until done"=FALSE ("结束前等待"), "Auto Dispose Ref"=FALSE ("自动销毁引用")) -> ()  [unwired: 2 in, 5 out]
        }
      }
    }
    frame Enabled {
    }
  }
  n308 = while {
    stop <- FALSE stop-if-true
    n309 = event shown="[2] \"IP1\", \"PORT1\", \"确定\": 值改变" {
      selector: _ -> [_ _ _ _ _ _ _ _ _ _ _ _]
      dyn-events: _ -> [_ _ _ _ _ _ _ _ _ _ _ _]
      timeout: _ -> [_ _ _ _ _ _ _ _ _ _ _ _]
      event Timeout {
        n310 = event-data() -> ()  [unwired: 1 in, 2 out]
      }
      event "站点名称", "IP", "port", "配置模式", "站点设备": Value Change {
        # "TCP服务器端口掉线"
        n311 = event-data() -> ()  [unwired: 1 in, 6 out]
        n312 = local read "线程选择"() -> (w355:string)
        n313 = case shown="\"线程一\", 默认" w355 {
          tunnel: ["线程一部署站点保存" "线程二部署站点保存" "线程三部署站点保存"] -> w354
          frame "线程一", Default {
          }
          frame "线程二" {
          }
          frame "线程三" {
          }
        }
        n314 = call <vilib>:"Application Directory.vi"() -> ("Application Directory"=w386:path)
        n315 = Build Path(base path=w386, name or relative path="data\\Set.ini" ("名称或相对路径")) -> (appended path=w384:path)
        n316 = local read "站点名称"() -> (w381:string)
        n317 = call <vilib>:"Open Config Data.vi"("configuration file path"=w384) -> ("error out"=w382:errorcluster, "refnum"=w383:T6)  [unwired: 8 in, 1 out]
        n318 = local read "站点设备"() -> (w376:string)
        n319 = call-poly <vilib>:"Write Key.vi"("section"=w354, "error in (no error)"=w382, "value"=w381, "key"="站点名称", "refnum"=w383) -> ("error out"=w378:errorcluster, "refnum out"=w379:T6)  [unwired: 4 in, 1 out]
        n320 = call-poly <vilib>:"Write Key.vi"("section"=w354, "error in (no error)"=w378, "value"=w376, "key"="站点设备", "refnum"=w379) -> ("error out"=w374:errorcluster, "refnum out"=w375:T6)  [unwired: 4 in, 1 out]
        n321 = local read "IP"() -> (w371:string)
        n322 = call-poly <vilib>:"Write Key.vi"("section"=w354, "error in (no error)"=w374, "value"=w371, "key"="IP", "refnum"=w375) -> ("error out"=w372:errorcluster, "refnum out"=w373:T6)  [unwired: 4 in, 1 out]
        n323 = local read "主队列输出"() -> (w363:refnum<queue>)
        n324 = local read "port"() -> (w370:string)
        n325 = local read "连接ID"() -> (w358:refnum<k5>)
        n326 = local read "配置模式"() -> (w369:u16)
        n327 = call-poly <vilib>:"Write Key.vi"("section"=w354, "error in (no error)"=w372, "value"=w370, "key"="PORT", "refnum"=w373) -> ("error out"=w366:errorcluster, "refnum out"=w367:T6)  [unwired: 4 in, 1 out]
        n328 = Flush Queue(queue=w363) -> (queue out=w362:refnum<queue>)  [unwired: 1 in, 2 out]
        n329 = TCP Close Connection(connection ID=w358) -> (error out=w359:errorcluster)  [unwired: 2 in, 1 out]
        n330 = call-poly <vilib>:"Write Key.vi"("section"=w354, "error in (no error)"=w366, "value"=w369, "key"="配置模式", "refnum"=w367) -> ("error out"=w364:errorcluster, "refnum out"=w365:T6)  [unwired: 4 in, 1 out]
        n331 = call <vilib>:"Clear Errors.vi"("error in (no error)"=w359) -> ()  [unwired: 5 in, 2 out]
        n332 = call <vilib>:"Close Config Data.vi"("error in (no error)"=w364, "refnum"=w365) -> ()  [unwired: 8 in, 2 out]
        n333 = Enqueue Element(queue=w362, element=T1."初始化" ("元素"), timeout in ms (-1)=1000 ("超时毫秒(-1)")) -> ()  [unwired: 1 in, 3 out]
      }
      event "IP1", "PORT1", "确定": Value Change {
        # "TCP服务器端口掉线"
        n334 = local read "线程选择"() -> (w391:string)
        n335 = event-data() -> ()  [unwired: 1 in, 6 out]
        n336 = case shown="\"线程一\", 默认" w391 {
          tunnel: ["线程一自主部署站点保存" "线程二自主部署站点保存" "线程三自主部署站点保存"] -> w390
          frame "线程一", Default {
          }
          frame "线程二" {
          }
          frame "线程三" {
          }
        }
        n337 = call <vilib>:"Application Directory.vi"() -> ("Application Directory"=w429:path)
        n338 = Build Path(base path=w429, name or relative path="data\\Set.ini" ("名称或相对路径")) -> (appended path=w427:path)
        n339 = local read "站点名称1"() -> (w424:string)
        n340 = call <vilib>:"Open Config Data.vi"("configuration file path"=w427) -> ("error out"=w425:errorcluster, "refnum"=w426:T6)  [unwired: 8 in, 1 out]
        n341 = local read "站点设备1"() -> (w419:string)
        n342 = call-poly <vilib>:"Write Key.vi"("section"=w390, "error in (no error)"=w425, "value"=w424, "key"="站点名称1", "refnum"=w426) -> ("error out"=w421:errorcluster, "refnum out"=w422:T6)  [unwired: 4 in, 1 out]
        n343 = call-poly <vilib>:"Write Key.vi"("section"=w390, "error in (no error)"=w421, "value"=w419, "key"="站点设备1", "refnum"=w422) -> ("error out"=w417:errorcluster, "refnum out"=w418:T6)  [unwired: 4 in, 1 out]
        n344 = local read "IP1"() -> (w412:string)
        n345 = local read "PORT1"() -> (w411:string)
        n346 = local read "主队列输出"() -> (w400:refnum<queue>)
        n347 = call-poly <vilib>:"Write Key.vi"("section"=w390, "error in (no error)"=w417, "value"=w412, "key"="IP1", "refnum"=w418) -> ("error out"=w415:errorcluster, "refnum out"=w416:T6)  [unwired: 4 in, 1 out]
        n348 = local read "MN1"() -> (w404:string)
        n349 = local read "连接ID"() -> (w395:refnum<k5>)
        n350 = call-poly <vilib>:"Write Key.vi"("section"=w390, "error in (no error)"=w415, "value"=w411, "key"="PORT1", "refnum"=w416) -> ("error out"=w407:errorcluster, "refnum out"=w408:T6)  [unwired: 4 in, 1 out]
        n351 = Flush Queue(queue=w400) -> (queue out=w399:refnum<queue>)  [unwired: 1 in, 2 out]
        n352 = TCP Close Connection(connection ID=w395) -> (error out=w396:errorcluster)  [unwired: 2 in, 1 out]
        n353 = call-poly <vilib>:"Write Key.vi"("section"=w390, "error in (no error)"=w407, "value"=w404, "key"="MN1", "refnum"=w408) -> ("error out"=w405:errorcluster, "refnum out"=w406:T6)  [unwired: 4 in, 1 out]
        n354 = call <vilib>:"Clear Errors.vi"("error in (no error)"=w396) -> ()  [unwired: 5 in, 2 out]
        n355 = local read "PW1"() -> (w403:string)
        n356 = call-poly <vilib>:"Write Key.vi"("section"=w390, "error in (no error)"=w405, "value"=w403, "key"="PW1", "refnum"=w406) -> ("error out"=w401:errorcluster, "refnum out"=w402:T6)  [unwired: 4 in, 1 out]
        n357 = Enqueue Element(queue=w399, element=T1."初始化" ("元素"), timeout in ms (-1)=1000 ("超时毫秒(-1)")) -> ()  [unwired: 1 in, 3 out]
        n358 = local read "配置模式"() -> (w394:u16)
        n359 = call <vilib>:"Close Config Data.vi"("error in (no error)"=w401, "refnum"=w402) -> ("error out"=w392:errorcluster)  [unwired: 8 in, 1 out]
        n360 = case shown="1" w394 {
          tunnel: [w437 w438] -> w393
          tunnel: w392 -> [w437 w438]
          frame 0, Default {
          }
          frame 1 {
            n361 = local read "IP1"() -> (w441:string)
            n362 = local read "站点名称1"() -> (w439:string)
            n363 = local read "PORT1"() -> (w442:string)
            n364 = local read "MN1"() -> (w443:string)
            n365 = local read "站点设备1"() -> (w440:string)
            n366 = local write "IP"(w441) -> ()
            n367 = local write "MN"(w443) -> ()
            n368 = local write "port"(w442) -> ()
            n369 = local read "PW1"() -> (w444:string)
            n370 = local write "站点名称"(w439) -> ()
            n371 = local write "站点设备"(w440) -> ()
            n372 = local write "PW"(w444) -> ()
          }
        }
        n373 = case shown="错误" w393 {
          frame No Error {
            n374 = One Button Dialog(message="保存成功" ("消息"), button name ("OK")="确定" ("按钮名称（“确定”）")) -> ()  [unwired: 1 out]
          }
          frame Error {
            n375 = One Button Dialog(message="保存失败" ("消息"), button name ("OK")="确定" ("按钮名称（“确定”）")) -> ()  [unwired: 1 out]
          }
        }
      }
      event "参数配置": Value Change {
        n376 = event-data() -> ()  [unwired: 1 in, 6 out]
        n377 = property on="窗格" class="Pane"("Origin"=T5 {"Horizontal"=0, "Vertical"=1000} ("原点")) -> ()  [unwired: 2 in, 2 out]
      }
      event "返回": Value Change {
        n378 = event-data() -> ()  [unwired: 1 in, 6 out]
        n379 = property on="窗格" class="Pane"("Origin"=T5 {"Horizontal"=0, "Vertical"=0} ("原点")) -> ()  [unwired: 2 in, 2 out]
      }
      event "系统编码选择框": Value Change {
        n380 = event-data() -> ()  [unwired: 1 in, 6 out]
        n381 = call <vilib>:"Application Directory.vi"() -> ("Application Directory"=w455:path)
        n382 = Build Path(base path=w455, name or relative path="data\\Set.ini" ("名称或相对路径")) -> (appended path=w456:path)
        n383 = call <vilib>:"Open Config Data.vi"("configuration file path"=w456) -> ("error out"=w452:errorcluster, "refnum"=w453:T6)  [unwired: 8 in, 1 out]
        n384 = call-poly <vilib>:"Write Key.vi"("section"="系统编码选择", "error in (no error)"=w452, "value"="系统编码选择框", "key"="系统编码", "refnum"=w453) -> ("error out"=w450:errorcluster, "refnum out"=w451:T6)  [unwired: 4 in, 1 out]
        n385 = call <vilib>:"Close Config Data.vi"("error in (no error)"=w450, "refnum"=w451) -> ()  [unwired: 8 in, 2 out]
      }
      event "站点名称1": Mouse Down {
        n386 = event-data() -> ()  [unwired: 1 in, 6 out]
        n387 = disable-structure shown="禁用" {
          frame Disabled {
            n388 = local read "站点名称1"() -> (w458:string)
            n389 = call "字符键盘.vi"("原值"=w458) -> ("x+y"=w457:string)  [unwired: 10 in]
            n390 = local write "站点名称1"(w457) -> ()
          }
          frame Enabled {
          }
        }
      }
      event "站点设备1": Mouse Down {
        n391 = event-data() -> ()  [unwired: 1 in, 6 out]
        n392 = disable-structure shown="禁用" {
          frame Disabled {
            n393 = local read "站点设备1"() -> (w460:string)
            n394 = call "字符键盘.vi"("原值"=w460) -> ("x+y"=w459:string)  [unwired: 10 in]
            n395 = local write "站点设备1"(w459) -> ()
          }
          frame Enabled {
          }
        }
      }
      event "IP1": Mouse Down {
        n396 = event-data() -> ()  [unwired: 1 in, 6 out]
        n397 = local read "IP1"() -> (w462:string)
        n398 = call "IP键盘.vi"("OldNumber"=w462) -> ("NewNumber"=w461:string)
        n399 = local write "IP1"(w461) -> ()
      }
      event "PORT1": Mouse Down {
        n400 = event-data() -> ()  [unwired: 1 in, 6 out]
        n401 = local read "PORT1"() -> (w464:string)
        n402 = call "IP键盘.vi"("OldNumber"=w464) -> ("NewNumber"=w463:string)
        n403 = local write "PORT1"(w463) -> ()
      }
      event "MN1": Mouse Down {
        n404 = event-data() -> ()  [unwired: 1 in, 6 out]
        n405 = local read "MN1"() -> (w466:string)
        n406 = call "字符键盘.vi"("原值"=w466) -> ("x+y"=w465:string)  [unwired: 10 in]
        n407 = local write "MN1"(w465) -> ()
      }
      event "PW1": Mouse Down {
        n408 = event-data() -> ()  [unwired: 1 in, 6 out]
        n409 = local read "PW1"() -> (w468:string)
        n410 = call "字符键盘.vi"("原值"=w468) -> ("x+y"=w467:string)  [unwired: 10 in]
        n411 = local write "PW1"(w467) -> ()
      }
    }
  }
  n412 = while {
    stop <- FALSE stop-if-true
    # "定期释放缓存"
    n413 = dll-call lib="PTH2_abs FSTD所有程序资料*平台数采程序 - 古田（2019.2.27）dataFreeMem.dll" fn="FreeMem"() -> ()  [unwired: 4 in, 2 out]
    n414 = Wait (ms)(milliseconds to wait=u32 600000 ("等待时间（毫秒）")) -> ()  [unwired: 1 out]
  }
  n415 = while {
    stop <- FALSE stop-if-true
    # "心跳包"
    n416 = global read "全局 数据发送重叠.vi" "掉线指示灯"() -> (→"掉线指示":bool)
    n417 = local read "IP"() -> (w480:string)
    n418 = local read "站点名称"() -> (w482:string)
    n419 = local read "MN"() -> (w478:string)
    n420 = local read "站点设备"() -> (w481:string)
    n421 = local read "port"() -> (w479:string)
    n422 = Get Date/Time In Seconds() -> (seconds since 1Jan1904=→"时间标识":timestamp)
    n423 = local read "PW"() -> (w477:string)
    n424 = Wait (ms)(milliseconds to wait=u32 1000 ("等待时间（毫秒）")) -> ()  [unwired: 1 out]
    n425 = local read "空闲时间"() -> (w495:dbl)
    n426 = local read "数据上传"() -> (w475:bool)
    n427 = Bundle By Name(cluster=T2 {"站点"="", "设备"="", "IP"="", "PORT"="", "MN"="", "PW"=""} ("配置信息"), "站点"=w482, "设备"=w481, "IP"=w480, "PORT"=w479, "MN"=w478, "PW"=w477) -> (→"配置信息":T2)
    n428 = case shown="0, 默认" "配置模式" {
      frame 0, Default {
        n429 = case shown="\"城东街道利洋村\"" "站点设备" {
          tunnel: ["82C18H003" ("设备编码MN") "82C18H005" ("设备编码MN") "82C18H001" ("设备编码MN") "82C18H002" ("设备编码MN") "82C18H004" ("设备编码MN") "82C18H006" ("设备编码MN") "82C18H007" ("设备编码MN") "82C18H008" ("设备编码MN") "82C18H009" ("设备编码MN") "82C18H010" ("设备编码MN") "82C18H011" ("设备编码MN") "82C18H012" ("设备编码MN") "82C18H013" ("设备编码MN") "82C18H014" ("设备编码MN") "82C18H015" ("设备编码MN") "82C18H016" ("设备编码MN") "82C18H017" ("设备编码MN") "82C18H018" ("设备编码MN") "82C18H019" ("设备编码MN") "82C18H020" ("设备编码MN") "82B18H019" ("设备编码MN") "82B18H020" ("设备编码MN") "82B18H021" ("设备编码MN") "82B18H022" ("设备编码MN") "82B18H023" ("设备编码MN") "82B18H024" ("设备编码MN") "TLHST0001" ("设备编码MN") "TLHST0002" ("设备编码MN") "TLHST0003" ("设备编码MN") "TLHST0004" ("设备编码MN") "34082332ZYWS02" ("设备编码MN") "34070032XMWS01" ("设备编码MN")] -> w500
          frame "凤埔乡平沙村", Default {
          }
          frame "凤埔乡苏墩村" {
          }
          frame "凤埔乡禾兴厂" {
          }
          frame "平湖镇定居坂" {
          }
          frame "平湖镇造粒厂" {
          }
          frame "平湖镇达才村" {
          }
          frame "平湖镇乔洋村" {
          }
          frame "平湖镇柏源溪口" {
          }
          frame "平湖镇溪州溪" {
          }
          frame "大桥镇横洋溪" {
          }
          frame "大桥镇瑞岩村村委" {
          }
          frame "大桥镇沽洋村" {
          }
          frame "吉巷乡渭洋溪" {
          }
          frame "吉巷乡前拢村" {
          }
          frame "吉巷乡韦端村" {
          }
          frame "城东街道利洋村" {
          }
          frame "城东街道常坝村" {
          }
          frame "城西街道龙亭村" {
          }
          frame "洋洋乡污水水厂" {
          }
          frame "黄田镇谷口大桥" {
          }
          frame "凤埔污水处理厂" {
          }
          frame "平湖污水处理厂" {
          }
          frame "大桥污水处理厂" {
          }
          frame "吉巷污水处理厂" {
          }
          frame "洋洋污水处理厂" {
          }
          frame "凤都污水处理厂" {
          }
          frame "铜陵二冶" {
          }
          frame "铜陵国电" {
          }
          frame "铜陵三厂" {
          }
          frame "铜陵城北" {
          }
          frame "铜陵枞阳" {
          }
          frame "铜陵新民" {
          }
        }
        n430 = local write "PW"("123456" ("密码PW")) -> ()
        n431 = local write "MN"(w500) -> ()
      }
      frame 1 {
        n432 = local read "IP1"() -> (w536:string)
        n433 = local read "站点名称1"() -> (w534:string)
        n434 = local read "PORT1"() -> (w537:string)
        n435 = local read "MN1"() -> (w538:string)
        n436 = local read "站点设备1"() -> (w535:string)
        n437 = local write "IP"(w536) -> ()
        n438 = local write "MN"(w538) -> ()
        n439 = local write "port"(w537) -> ()
        n440 = local read "PW1"() -> (w539:string)
        n441 = local write "站点名称"(w534) -> ()
        n442 = local write "站点设备"(w535) -> ()
        n443 = local write "PW"(w539) -> ()
      }
    }
    n444 = local read "步骤"() -> (w489:T1)
    n445 = local read "系统编码选择框"() -> (w472:string)
    n446 = Greater?(x=w495, y=30.0) -> (0:w493:bool)
    n447 = Not(x=w475) -> (.not. x?=w474:bool)
    n448 = Equal?(x=w489, y=T1."读取数据" ("步骤")) -> (x = y?=w487:bool)
    n449 = case shown="真" w493 {
      tunnel: w493 -> [_ w545]
      tunnel: [FALSE w545] -> w490
      frame False {
      }
      frame True {
        w544 = 0.0 ("空闲时间")
        n450 = local write "try"(w544) -> ()
        n451 = local read "MN"() -> (w547:string)
        n452 = local read "QN"() -> (w542:string)
        n453 = local read "PW"() -> (w546:string)
        n454 = local write "空闲时间"(w544) -> ()
        n455 = local read "连接ID"() -> (w549:refnum<k5>)
        n456 = call "数据编码.vi"("table输入"="心跳包", "QN"=w542, "MN"=w547, "PW"=w546) -> ("通讯包字符串"=w541:string)  [unwired: 10 in, 1 out]
        n457 = local write "发送报文显示"(w541) -> ()
        n458 = TCP Write(connection ID=w549, data in=w541) -> (error out=w543:errorcluster)  [unwired: 2 in, 2 out]
        n459 = call <vilib>:"Clear Errors.vi"("error in (no error)"=w543) -> ()  [unwired: 5 in, 2 out]
      }
    }
    "心跳包" <- w490
    n460 = Or(x=w487, y=w474) -> (x .or. y?=w476:bool)
    n461 = case shown="真" w476 {
      frame False {
        n462 = local write "空闲时间"(0.0 ("空闲时间")) -> ()
      }
      frame True {
        n463 = local read "空闲时间"() -> (w552:dbl)
        n464 = Increment(x=w552) -> (x+1=→"空闲时间":dbl)
      }
    }
    n465 = case shown="\"地表水质量监测\", 默认" w472 {
      tunnel: ["52" ("设备编码MN") "32" ("设备编码MN") "21" ("设备编码MN")] -> w471
      frame "污水排放过程监测" {
      }
      frame "地表水体污染源" {
      }
      frame "地表水质量监测", Default {
      }
    }
    n466 = global write "全局1.vi" "系统编码ST"(w471) -> ()
  }
  n467 = for {
    N: 1 -> [_]
    w623 = "" ("参数")
    w574 = FALSE ("数据发送中断")
    w637 = 0.0 ("try")
    # "ST参数选择"
    # "初始化"
    n468 = property class="VI"() -> ("Panel"=w628:refnum<vi>)  [unwired: 2 in, 2 out]
    n469 = case shown="\"线程一\", 默认" "线程选择" {
      tunnel: ["线程一部署站点保存" "线程二部署站点保存" "线程三部署站点保存"] -> w560
      frame "线程一", Default {
      }
      frame "线程二" {
      }
      frame "线程三" {
      }
    }
    n470 = local write "心跳包"(FALSE ("心跳包")) -> ()
    n471 = local write "数据接收中断"(FALSE ("数据发送中断")) -> ()
    n472 = global write "全局 小时数据发送次数.vi" "小时数据发送次数"(0 ("数值")) -> ()
    n473 = property class="Pnl"(reference=w628) -> ("Panes[]"=w627:refnum<vi>[])  [unwired: 1 in, 2 out]
    n474 = global write "全局 实时数据参数.vi" "data"(string[][] [] ("data")) -> ()
    n475 = global write "全局 实时数据参数.vi" "参数"(w623) -> ()
    n476 = local write "try"(w637) -> ()
    n477 = property on="窗格" class="Pane"("Origin"=T5 {"Horizontal"=0, "Vertical"=0} ("原点")) -> ()  [unwired: 2 in, 2 out]
    n478 = local write "数据正在发送"(w574) -> ()
    n479 = local write "重发数据"(w574) -> ()
    n480 = local write "空闲时间"(w637) -> ()
    n481 = global write "全局 实时数据参数.vi" "连接的字符串"(w623) -> ()
    n482 = local write "数据上传"(w574) -> ()
    n483 = call <vilib>:"Application Directory.vi"() -> ("Application Directory"=w621:path)
    n484 = for {
      tunnel: w627 -> [w645] mode=indexing
      tunnel: u32 15592941 ("窗格颜色") -> [w646]
      n485 = property class="Pane"(reference=w645, "PaneColor"=w646) -> ()  [unwired: 1 in, 2 out]
    }
    n486 = global write "全局1.vi" "枚举"(enum16{"返回请求应答", "上传数据", "返回执行结果"}."返回请求应答" ("枚举")) -> ()
    n487 = Build Path(base path=w621, name or relative path="data\\Set.ini" ("名称或相对路径")) -> (appended path=w619:path)
    n488 = call <vilib>:"Open Config Data.vi"("configuration file path"=w619) -> ("error out"=w617:errorcluster, "refnum"=w618:T6)  [unwired: 8 in, 1 out]
    n489 = Get Date/Time In Seconds() -> (seconds since 1Jan1904=w632:timestamp)
    n490 = Format Date/Time String(time format string (%c)="%Y%m%d%H%M%S%3u" ("时间格式字符串(%c)"), seconds (now)=w632) -> (date/time string=w631:string)  [unwired: 1 in]
    n491 = call-poly <vilib>:"Read Key.vi"("section"=w560, "error in (no error)"=w617, "key"="站点名称", "refnum"=w618) -> ("error out"=w613:errorcluster, "value"=w615:string, "refnum out"=w614:T6)  [unwired: 4 in, 1 out]
    n492 = control-ref of="本VI"() -> (w557:refnum<vi>)
    n493 = local write "站点名称"(w615) -> ()
    n494 = Search and Replace String(input string=w631, search string="." ("搜索字符串")) -> (result string=w629:string)  [unwired: 6 in, 3 out]
    n495 = property class="VI"(reference=w557) -> ("Hist.Revision"=w556:u32)  [unwired: 1 in, 2 out]
    n496 = local write "QN"(w629) -> ()
    n497 = call-poly <vilib>:"Read Key.vi"("section"=w560, "error in (no error)"=w613, "key"="站点设备", "refnum"=w614) -> ("error out"=w609:errorcluster, "value"=w611:string, "refnum out"=w610:T6)  [unwired: 4 in, 1 out]
    n498 = Number To Decimal String(number=w556) -> (decimal integer string=w555:string)  [unwired: 1 in]
    n499 = local write "站点设备"(w611) -> ()
    n500 = local read "线程选择"() -> (w559:string)
    n501 = Concatenate Strings("20190228V4.5." ("软件版本"), w555) -> (→"软件版本":string)
    n502 = call-poly <vilib>:"Read Key.vi"("section"=w560, "error in (no error)"=w609, "key"="IP", "refnum"=w610) -> ("error out"=w605:errorcluster, "value"=w607:string, "refnum out"=w606:T6)  [unwired: 4 in, 1 out]
    n503 = case shown="\"线程一\", 默认" w559 {
      tunnel: ["线程一自主部署站点保存" "线程二自主部署站点保存" "线程三自主部署站点保存"] -> w558
      frame "线程一", Default {
      }
      frame "线程二" {
      }
      frame "线程三" {
      }
    }
    n504 = local write "IP"(w607) -> ()
    n505 = call-poly <vilib>:"Read Key.vi"("section"=w560, "error in (no error)"=w605, "key"="PORT", "refnum"=w606) -> ("error out"=w600:errorcluster, "value"=w603:string, "refnum out"=w601:T6)  [unwired: 4 in, 1 out]
    n506 = local write "port"(w603) -> ()
    n507 = call-poly <vilib>:"Read Key.vi"("section"=w560, "error in (no error)"=w600, "key"="配置模式", "refnum"=w601) -> ("error out"=w598:errorcluster, "value"=w599:i32, "refnum out"=w597:T6)  [unwired: 4 in, 1 out]
    n508 = local write "配置模式"(w599) -> ()
    n509 = call-poly <vilib>:"Read Key.vi"("section"=w558, "error in (no error)"=w598, "key"="站点名称1", "refnum"=w597) -> ("error out"=w593:errorcluster, "value"=w595:string, "refnum out"=w594:T6)  [unwired: 4 in, 1 out]
    n510 = local write "站点名称1"(w595) -> ()
    n511 = call-poly <vilib>:"Read Key.vi"("section"=w558, "error in (no error)"=w593, "key"="站点设备1", "refnum"=w594) -> ("error out"=w591:errorcluster, "value"=w589:string, "refnum out"=w592:T6)  [unwired: 4 in, 1 out]
    n512 = local write "站点设备1"(w589) -> ()
    n513 = call-poly <vilib>:"Read Key.vi"("section"=w558, "error in (no error)"=w591, "key"="IP1", "refnum"=w592) -> ("error out"=w587:errorcluster, "value"=w585:string, "refnum out"=w588:T6)  [unwired: 4 in, 1 out]
    n514 = local write "IP1"(w585) -> ()
    n515 = call-poly <vilib>:"Read Key.vi"("section"=w558, "error in (no error)"=w587, "key"="PORT1", "refnum"=w588) -> ("error out"=w581:errorcluster, "value"=w583:string, "refnum out"=w582:T6)  [unwired: 4 in, 1 out]
    n516 = local write "PORT1"(w583) -> ()
    n517 = call-poly <vilib>:"Read Key.vi"("section"=w558, "error in (no error)"=w581, "key"="MN1", "refnum"=w582) -> ("error out"=w579:errorcluster, "value"=w576:string, "refnum out"=w580:T6)  [unwired: 4 in, 1 out]
    n518 = local write "MN1"(w576) -> ()
    n519 = call-poly <vilib>:"Read Key.vi"("section"=w558, "error in (no error)"=w579, "key"="PW1", "refnum"=w580) -> ("error out"=w572:errorcluster, "value"=w575:string, "refnum out"=w573:T6)  [unwired: 4 in, 1 out]
    n520 = local write "PW1"(w575) -> ()
    n521 = call-poly <vilib>:"Read Key.vi"("section"="系统编码选择", "error in (no error)"=w572, "key"="系统编码", "refnum"=w573) -> ("error out"=w567:errorcluster, "value"=w569:string, "refnum out"=w568:T6)  [unwired: 4 in, 1 out]
    n522 = local write "系统编码选择框"(w569) -> ()
    n523 = call-poly <vilib>:"Read Key.vi"("section"="掉线时间存储", "error in (no error)"=w567, "key"="掉线时间", "refnum"=w568) -> ("error out"=w562:errorcluster, "value"=w564:string, "refnum out"=w563:T6)  [unwired: 4 in, 1 out]
    n524 = global write "全局 数据发送重叠.vi" "TCP掉线时间节点"(w564) -> ()
    n525 = local write "TCP掉线时间节点"(w564) -> ()
    n526 = call <vilib>:"Close Config Data.vi"("error in (no error)"=w562, "refnum"=w563) -> ()  [unwired: 8 in, 2 out]
    "TCP服务端掉线计数" <- 0
  }
  n527 = call "获取需发送的数据表.vi"() -> ("error out"=w38:errorcluster, "tables"=w47:string[])  [unwired: 10 in]
  n528 = call <vilib>:"Clear Errors.vi"("error in (no error)"=w38) -> ()  [unwired: 5 in, 2 out]
  n529 = property class="App"() -> ("App.Kind"=w30:T7)  [unwired: 2 in, 2 out]
  n530 = Insert Into Array(array=w47, index=0 ("索引"), new element="实时数据" ("新元素/子数组")) -> (w48:string[])
  n531 = case shown="\"Development System\", 默认" w30 {
    tunnel: [T8."Standard" ("状态") T8."Hidden" ("状态")] -> w3
    frame "Development System", Default {
    }
    frame "Run Time System" {
    }
  }
  n532 = call <vilib>:"Application Directory.vi"() -> ("Application Directory"=w24:path)
  n533 = Build Path(base path=w24, name or relative path="data\\tubiao.ico" ("名称或相对路径")) -> (appended path=w14:path)
  n534 = Array Size(array=w48) -> (size(s)=w45:i32)
  n535 = Current VI's Path() -> (path=w27:path)
  n536 = Build Array(w14) -> (w19:path[])
  n537 = Open VI Reference(vi path=w27) -> (vi reference=w28:refnum<vi>)  [unwired: 5 in, 1 out]
  n538 = invoke class="VI" method="FP.Open"(reference=w28, "Activate"=TRUE ("激活？"), "State"=w3) -> (error out=w29:errorcluster)  [unwired: 2 in, 4 out]
  n539 = call <vilib>:"Constructor.vi"("error in"=w29, "IconFilePathList"=w19) -> ("error out"=w15:errorcluster, "NotifyIcon"=w23:refnum<class "NotifyIcon.lvclass">)  [unwired: 8 in]
  n540 = Obtain Queue(name (unnamed)="STEP" ("名称（未命名）"), element data type=T1."初始化" ("枚举")) -> (queue out=w43:refnum<queue>)  [unwired: 3 in, 2 out]
  n541 = for {
    shift-right: [w653] -> w1
    shift-left: w15 -> [w654]
    tunnel: string[] ["Open线程二", "-", "Exit线程二"] -> [w652] mode=indexing
    tunnel: w22 -> [w651] mode=indexing
    shift-right: [w649] -> w2
    shift-left: w23 -> [w650]
    # "2."
    n542 = call <vilib>:"InsertMenuItem.vi"("error in"=w654, "ItemTag"=w651, "ItemName"=w652, "NotifyIcon in"=w650) -> ("error out"=w653:errorcluster, "NotifyIcon out"=w649:refnum<class "NotifyIcon.lvclass">)  [unwired: 6 in]
  }
  n543 = Index Array(array=w22) -> (element=w21:string)  [unwired: 1 in]
  n544 = Enqueue Element(queue=w43, element=T1."初始化" ("元素")) -> (queue out=w52:refnum<queue>)  [unwired: 2 in, 2 out]
  "主队列输出" <- w52
  n545 = property class="NotifyIcon"(reference=w2, error in=w1, "Public:Visible"=TRUE ("Visible"), "Public:DefaultMenuItem"=w21, "Public:TipText"="平台发送系统线程二" ("TipText")) -> (reference out=w7:refnum<class "NotifyIcon.lvclass">, error out=w16:errorcluster, "Public:SelectedItemEvent"=w17:refnum<user-event>)
  n546 = while {
    shift-right: [w656] -> _
    shift-left: errorcluster {"status"=FALSE, "code"=0, "source"=""} ("error out") -> [w670]
    shift-right: [w660] -> _
    shift-left: refnum<k5> refnum ("connection ID") -> [w661]
    shift-right: [w667] -> _
    shift-left: _ -> [w666]
    tunnel: w52 -> [w669]
    tunnel: w48 -> [w665]
    shift-right: [w663] -> _
    shift-left: 0 ("索引") -> [w664]
    tunnel: w45 -> [w662]
    shift-right: [w658] -> _
    shift-left: 0 ("索引") -> [w659]
    i -> [w655]
    stop <- FALSE stop-if-true
    n547 = Wait (ms)(milliseconds to wait=u32 300 ("等待时间（毫秒）")) -> ()  [unwired: 1 out]
    n548 = case shown="无错误" w670 {
      selector: w670 -> [w689 w1267]
      tunnel: w661 -> [w690 w1273]
      tunnel: [w685 w1272] -> w660
      tunnel: [w671 w1270] -> w656
      tunnel: w669 -> [w688 w1265]
      tunnel: [w672 w1269] -> w667
      tunnel: w666 -> [w684 w1269]
      tunnel: w665 -> [w683 _]
      tunnel: w664 -> [w678 w1268]
      tunnel: [w681 w1268] -> w663
      tunnel: w662 -> [w680 _]
      tunnel: w659 -> [w675 w1264]
      tunnel: [w674 w1264] -> w658
      frame No Error {
        n549 = Less?(x=w678, y=w680) -> (x < y?=w679:bool)
        n550 = Dequeue Element(queue=w688) -> (queue out=w686:refnum<queue>, element=w687:T1)  [unwired: 2 in, 2 out]
        "步骤" <- w687
        n551 = Select(t=w678, s=w679, f=0) -> (s? t:f=w677:i32)
        n552 = local read "元素"() -> (w673:string)
        n553 = Index Array(array=w683, index=w677) -> (element=→"元素":string)
        n554 = case shown="\"读取数据\"" w687 {
          tunnel: w690 -> [w697 _ w731 w892 w1182 w1261]
          tunnel: w689 -> [w698 _ w730 w897 w1178 w1260]
          tunnel: w686 -> [w693 w710 w721 w867 w1175 w1258]
          tunnel: [w698 w699 w730 w863 w1174 w1260] -> w671
          tunnel: [w697 w703 w731 w893 w1179 w1261] -> w685
          tunnel: [string[] [] ("待发送第一条数据") w712 w717 w891 w1180 _] -> w672
          tunnel: w684 -> [_ w712 _ w891 w1180 w1259]
          tunnel: w673 -> [_ _ _ _ _ w1252]
          tunnel: w677 -> [w694 w709 w725 w895 w1181 w1248]
          tunnel: [w694 w709 w724 w895 w1181 w1249] -> w681
          tunnel: w675 -> [w691 w707 w723 _ w1170 w1246]
          tunnel: [w691 w707 w723 0 ("索引") w1173 w1246] -> w674
          frame "初始化", Default {
            n555 = Enqueue Element(queue=w693, element=T1."打开连接" ("元素"), timeout in ms (-1)=1000 ("超时毫秒(-1)")) -> ()  [unwired: 1 in, 3 out]
          }
          frame "打开连接" {
            (unwired) "47.98.43.76"
            # "和时通数据接入平台端接收IP端口号，61.191.22.195:10003。"
            # "47.98.43.76:6666"
            n556 = Enqueue Element(queue=w710, element=T1."表格比对" ("元素"), timeout in ms (-1)=1000 ("超时毫秒(-1)")) -> ()  [unwired: 1 in, 3 out]
            n557 = Decimal String To Number(string="port") -> (number=w704:i32)  [unwired: 2 in, 1 out]
            n558 = TCP Open Connection(address="IP", remote port or service name=w704) -> (connection ID=w703:refnum<k5>, error out=w699:errorcluster)  [unwired: 3 in]
            n559 = local write "连接ID"(w703) -> ()
            n560 = Unbundle By Name(w699) -> ("status"=w701:bool, "code"=→"1st Error to Convert":i32)
            n561 = Not(x=w701) -> (.not. x?=→"通信状态":bool)
          }
          frame "表格比对" {
            # "在发送数据完之后通过TCP掉线计数仍然大于1且列队中还有元素判定再次回到表格对比\n再在表格对比这里加上出列队（前提先一次把水样测试、核查等5个元素入列队）...........LOOP直到5种测量数据全部发送完毕"
            n562 = local read "TCP服务端掉线计数"() -> (w716:i32)
            n563 = Greater Or Equal?(x=w716, y=1) -> (x >= y?=w713:bool)
            n564 = case shown="真" w713 {
              tunnel: [T1."读取数据" ("元素") w733] -> w714
              frame False {
              }
              frame True {
                n565 = local read "重发数据"() -> (w734:bool)
                n566 = Obtain Queue(name (unnamed)="重发掉线数据" ("名称（未命名）"), element data type=T9."水样测试") -> (queue out=w740:refnum<queue>, error out=w737:errorcluster)  [unwired: 3 in, 1 out]
                n567 = case shown="假" w734 {
                  tunnel: w740 -> [w746 w753]
                  tunnel: [w744 w753] -> w738
                  tunnel: w737 -> [w743 w752]
                  tunnel: [w742 w752] -> w736
                  frame False {
                    n568 = for {
                      N: 8 -> [_]
                      tunnel: w746 -> [w751]
                      tunnel: [w749] -> w744
                      tunnel: w743 -> [w748]
                      tunnel: [w747] -> w742
                      i -> [w750]
                      n569 = Enqueue Element(queue=w751, element=w750, error in (no error)=w748) -> (queue out=w749:refnum<queue>, error out=w747:errorcluster)  [unwired: 1 in, 1 out]
                    }
                  }
                  frame True {
                  }
                }
                n570 = Dequeue Element(queue=w738, error in (no error)=w736) -> (element=w735:T9)  [unwired: 1 in, 3 out]
                n571 = case shown="\"水样测试\", 默认" w735 {
                  tunnel: [w754 w769 w783 w793 w803 w816 w829 w842] -> w733
                  frame "水样测试", Default {
                    n572 = flat-sequence {
                      tunnel: [w762] -> w754
                      frame #0 {
                        n573 = global write "全局 小时数据发送次数.vi" "小时数据发送次数"(0 ("数值")) -> ()
                        n574 = global write "全局 实时数据参数.vi" "实时数据参数"("水样测试") -> ()
                        n575 = local write "table元素"("提取实时数据" ("新元素/子数组")) -> ()
                        n576 = global write "全局1.vi" "枚举"(enum16{"返回请求应答", "上传数据", "返回执行结果"}."上传数据" ("枚举")) -> ()
                      }
                      frame #1 {
                        n577 = call "从数据库获取数据通用可配置(子VI).vi"("table输入"="实时数据" ("新元素/子数组"), "列队名（唯一）"="adiao") -> ()  [unwired: 8 in, 2 out]
                      }
                      frame #2 {
                        # "数据处理整合"
                        n578 = call "数据处理整合 (子VI).vi"("枚举"=enum16{"实时数据排序", "小时数据排序"}."实时数据排序") -> ("已排序的数组"=w766:string[])  [unwired: 10 in]
                        n579 = Array Size(array=w766) -> (size(s)=w765:i32)
                        n580 = global write "全局 数据数组大小.vi" "数据数组大小"(w765) -> ()
                        n581 = Greater Than 0?(x=w765) -> (x > 0?=w764:bool)
                        n582 = case shown="真" w764 {
                          tunnel: [T1."表格比对" ("元素") T1."发送数据" ("元素")] -> w762
                          frame False {
                          }
                          frame True {
                          }
                        }
                        "重发数据" <- TRUE ("重发数据中")
                      }
                    }
                  }
                  frame "小时数据" {
                    n583 = flat-sequence {
                      tunnel: [w777] -> w769
                      frame #0 {
                        n584 = local read "TCP掉线时间节点"() -> (w771:string)
                        n585 = call "当前时间格式显示 (子VI).vi"() -> ("当前时间格式显示"=w770:string)  [unwired: 11 in]
                        n586 = global write "全局 时间2.vi" "小时数据时间2"(w770) -> ()
                        n587 = global write "全局 时间.vi" "小时数据时间"(w771) -> ()
                        n588 = global write "全局 小时数据发送次数.vi" "小时数据发送次数"(0 ("数值")) -> ()
                        n589 = local write "table元素"("小时数据" ("新元素/子数组")) -> ()
                        n590 = global write "全局1.vi" "枚举"(enum16{"返回请求应答", "上传数据", "返回执行结果"}."返回请求应答" ("枚举")) -> ()
                      }
                      frame #1 {
                        n591 = call "从数据库获取数据通用可配置(子VI).vi"("table输入"="小时数据" ("新元素/子数组"), "列队名（唯一）"="XS" ("名称（未命名）")) -> ()  [unwired: 8 in, 2 out]
                      }
                      frame #2 {
                        # "数据处理整合"
                        n592 = call "数据处理整合 (子VI).vi"() -> ("已排序的数组"=w780:string[])  [unwired: 11 in]
                        n593 = Array Size(array=w780) -> (size(s)=w779:i32)
                        n594 = global write "全局 数据数组大小.vi" "数据数组大小"(w779) -> ()
                        n595 = Greater Than 0?(x=w779) -> (x > 0?=w778:bool)
                        n596 = case shown="假" w778 {
                          tunnel: [T1."表格比对" ("元素") T1."发送数据" ("元素")] -> w777
                          frame False {
                          }
                          frame True {
                          }
                        }
                      }
                    }
                  }
                  frame "日志信息" {
                    n597 = flat-sequence {
                      tunnel: [w787] -> w783
                      frame #0 {
                        n598 = global write "全局 小时数据发送次数.vi" "小时数据发送次数"(0 ("数值")) -> ()
                        n599 = global write "全局1.vi" "枚举"(enum16{"返回请求应答", "上传数据", "返回执行结果"}."上传数据" ("枚举")) -> ()
                        n600 = local write "table元素"("操作日志" ("新元素/子数组")) -> ()
                      }
                      frame #1 {
                        n601 = call "获取操作日志 (子VI).vi"() -> ()  [unwired: 12 in]
                      }
                      frame #2 {
                        # "数据处理整合"
                        n602 = call "数据处理整合 (子VI).vi"() -> ("已排序的数组"=w790:string[])  [unwired: 11 in]
                        n603 = Array Size(array=w790) -> (size(s)=w789:i32)
                        n604 = global write "全局 数据数组大小.vi" "数据数组大小"(w789) -> ()
                        n605 = Greater Than 0?(x=w789) -> (x > 0?=w788:bool)
                        n606 = case shown="假" w788 {
                          tunnel: [T1."表格比对" ("元素") T1."发送数据" ("元素")] -> w787
                          frame False {
                          }
                          frame True {
                          }
                        }
                      }
                    }
                  }
                  frame "报警信息" {
                    n607 = flat-sequence {
                      tunnel: [w797] -> w793
                      frame #0 {
                        n608 = global write "全局 小时数据发送次数.vi" "小时数据发送次数"(0 ("数值")) -> ()
                        n609 = global write "全局1.vi" "枚举"(enum16{"返回请求应答", "上传数据", "返回执行结果"}."上传数据" ("枚举")) -> ()
                        n610 = local write "table元素"("报警信息" ("新元素/子数组")) -> ()
                      }
                      frame #1 {
                        n611 = call "获取报警信息 (子VI).vi"() -> ()  [unwired: 12 in]
                      }
                      frame #2 {
                        # "数据处理整合"
                        n612 = call "数据处理整合 (子VI).vi"() -> ("已排序的数组"=w800:string[])  [unwired: 11 in]
                        n613 = Array Size(array=w800) -> (size(s)=w799:i32)
                        n614 = Greater Than 0?(x=w799) -> (x > 0?=w798:bool)
                        n615 = global write "全局 数据数组大小.vi" "数据数组大小"(w799) -> ()
                        n616 = case shown="假" w798 {
                          tunnel: [T1."表格比对" ("元素") T1."发送数据" ("元素")] -> w797
                          frame False {
                          }
                          frame True {
                          }
                        }
                      }
                    }
                  }
                  frame "零点核查" {
                    n617 = flat-sequence {
                      tunnel: [w810] -> w803
                      frame #0 {
                        n618 = global write "全局 小时数据发送次数.vi" "小时数据发送次数"(0 ("数值")) -> ()
                        n619 = global write "全局 实时数据参数.vi" "实时数据参数"("空白测试") -> ()
                        n620 = local write "table元素"("实时数据" ("新元素/子数组")) -> ()
                        n621 = global write "全局1.vi" "枚举"(enum16{"返回请求应答", "上传数据", "返回执行结果"}."返回请求应答" ("枚举")) -> ()
                      }
                      frame #1 {
                        n622 = call "从数据库获取数据通用可配置(子VI).vi"("table输入"="实时数据" ("新元素/子数组"), "列队名（唯一）"="bdiao") -> ()  [unwired: 8 in, 2 out]
                      }
                      frame #2 {
                        # "数据处理整合"
                        n623 = call "数据处理整合 (子VI).vi"() -> ("已排序的数组"=w813:string[])  [unwired: 11 in]
                        n624 = Array Size(array=w813) -> (size(s)=w812:i32)
                        n625 = global write "全局 数据数组大小.vi" "数据数组大小"(w812) -> ()
                        n626 = Greater Than 0?(x=w812) -> (x > 0?=w811:bool)
                        n627 = case shown="假" w811 {
                          tunnel: [T1."表格比对" ("元素") T1."发送数据" ("元素")] -> w810
                          frame False {
                          }
                          frame True {
                          }
                        }
                      }
                    }
                  }
                  frame "标样核查" {
                    n628 = flat-sequence {
                      tunnel: [w823] -> w816
                      frame #0 {
                        n629 = global write "全局 小时数据发送次数.vi" "小时数据发送次数"(0 ("数值")) -> ()
                        n630 = global write "全局 实时数据参数.vi" "实时数据参数"("跨度核查") -> ()
                        n631 = global write "全局1.vi" "枚举"(enum16{"返回请求应答", "上传数据", "返回执行结果"}."返回请求应答" ("枚举")) -> ()
                        n632 = local write "table元素"("实时数据" ("新元素/子数组")) -> ()
                      }
                      frame #1 {
                        n633 = call "从数据库获取数据通用可配置(子VI).vi"("table输入"="实时数据" ("新元素/子数组"), "列队名（唯一）"="cdiao") -> ()  [unwired: 8 in, 2 out]
                      }
                      frame #2 {
                        # "数据处理整合"
                        n634 = call "数据处理整合 (子VI).vi"() -> ("已排序的数组"=w826:string[])  [unwired: 11 in]
                        n635 = Array Size(array=w826) -> (size(s)=w825:i32)
                        n636 = global write "全局 数据数组大小.vi" "数据数组大小"(w825) -> ()
                        n637 = Greater Than 0?(x=w825) -> (x > 0?=w824:bool)
                        n638 = case shown="假" w824 {
                          tunnel: [T1."表格比对" ("元素") T1."发送数据" ("元素")] -> w823
                          frame False {
                          }
                          frame True {
                          }
                        }
                      }
                    }
                  }
                  frame "平行样" {
                    n639 = flat-sequence {
                      tunnel: [w836] -> w829
                      frame #0 {
                        n640 = global write "全局 小时数据发送次数.vi" "小时数据发送次数"(0 ("数值")) -> ()
                        n641 = global write "全局 实时数据参数.vi" "实时数据参数"("平行样测试") -> ()
                        n642 = local write "table元素"("提取实时数据" ("新元素/子数组")) -> ()
                        n643 = global write "全局1.vi" "枚举"(enum16{"返回请求应答", "上传数据", "返回执行结果"}."上传数据" ("枚举")) -> ()
                      }
                      frame #1 {
                        n644 = call "从数据库获取数据通用可配置(子VI).vi"("table输入"="实时数据" ("新元素/子数组"), "列队名（唯一）"="ddiao") -> ()  [unwired: 8 in, 2 out]
                      }
                      frame #2 {
                        # "数据处理整合"
                        n645 = call "数据处理整合 (子VI).vi"() -> ("已排序的数组"=w839:string[])  [unwired: 11 in]
                        n646 = Array Size(array=w839) -> (size(s)=w838:i32)
                        n647 = global write "全局 数据数组大小.vi" "数据数组大小"(w838) -> ()
                        n648 = Greater Than 0?(x=w838) -> (x > 0?=w837:bool)
                        n649 = case shown="假" w837 {
                          tunnel: [T1."表格比对" ("元素") T1."发送数据" ("元素")] -> w836
                          frame False {
                          }
                          frame True {
                          }
                        }
                      }
                    }
                  }
                  frame "加标回收" {
                    n650 = flat-sequence {
                      tunnel: [w850] -> w842
                      frame #0 {
                        n651 = global write "全局 小时数据发送次数.vi" "小时数据发送次数"(0 ("数值")) -> ()
                        n652 = global write "全局 实时数据参数.vi" "实时数据参数"("加标回收测试") -> ()
                        n653 = global write "全局1.vi" "枚举"(enum16{"返回请求应答", "上传数据", "返回执行结果"}."上传数据" ("枚举")) -> ()
                        n654 = local write "table元素"("实时数据" ("新元素/子数组")) -> ()
                      }
                      frame #1 {
                        n655 = call "从数据库获取数据通用可配置(子VI).vi"("table输入"="加标回收" ("新元素/子数组"), "列队名（唯一）"="ediao") -> ()  [unwired: 8 in, 2 out]
                      }
                      frame #2 {
                        # "数据处理整合"
                        n656 = call "加标回收数据处理整合 (子VI).vi"() -> ("已排序的数组"=w849:string[])  [unwired: 11 in]
                        n657 = Array Size(array=w849) -> (size(s)=w852:i32)
                        n658 = global write "全局 数据数组大小.vi" "数据数组大小"(w852) -> ()
                        n659 = Greater Than 0?(x=w852) -> (x > 0?=w851:bool)
                        n660 = case shown="假" w851 {
                          tunnel: [T1."读取数据" ("元素") T1."发送数据" ("元素")] -> w850
                          frame False {
                          }
                          frame True {
                          }
                        }
                      }
                    }
                  }
                }
              }
            }
            n661 = call "数据表比对.vi"("查询元素输入"="氨氮" ("table输入 2"), "table输入"="实时数据") -> ("待发送第一条数据"=w717:string[], "待发送数据"=w718:string[][])  [unwired: 6 in, 2 out]
            n662 = Empty Array?(array=w718) -> (empty?=w729:bool)
            n663 = local read "心跳包"() -> (w726:bool)
            n664 = Not(x=w729) -> (.not. x?=w728:bool)
            n665 = Or(x=w728, y=w726) -> (x .or. y?=w727:bool)
            n666 = case shown="假" w727 {
              tunnel: w725 -> [w856 w857]
              tunnel: [w855 w857] -> w724
              frame False {
                n667 = Increment(x=w856) -> (x+1=w855:i32)
              }
              frame True {
              }
            }
            n668 = Enqueue Element(queue=w721, element=w714, timeout in ms (-1)=1000 ("超时毫秒(-1)")) -> ()  [unwired: 1 in, 3 out]
          }
          frame "读取数据" {
            w860 = FALSE ("数据正在发送")
            # "1000设置超时时间和重发次数\n1011提取监测仪表时间\n1012设置监测仪表时间\n1014提取数采仪时间\n1015设置数采仪时间\n1061提取实时数据间隔\n1062设置实时数据间隔\n1072设置数采仪访问密码"
            # "6分钟掉线重连"
            n669 = property on="TCP服务端掉线计数" class="DigNum (严格)"("Value"=0 ("TCP服务端掉线计数")) -> ()  [unwired: 2 in, 2 out]
            n670 = global write "全局 数据发送重叠.vi" "掉线指示灯"(FALSE ("数据发送重叠")) -> ()
            n671 = local write "重发数据"(w860) -> ()
            n672 = local write "数据正在发送"(w860) -> ()
            n673 = property on="实时数据发送时间间隔/min" class="DigNum (严格)"() -> ("Value"=w876:u32)  [unwired: 2 in, 2 out]
            n674 = global write "实时数据发送间隔全局.vi" "实时数据发送间隔"(w876) -> ()
            n675 = property on="设置超时时间/min" class="DigNum (严格)"() -> ("Value"=w879:i32)  [unwired: 2 in, 2 out]
            n676 = Multiply(x=w879, y=10000) -> (x*y=w877:i32)
            n677 = TCP Read(connection ID=w892, bytes to read=1024 ("读取的字节"), error in (no error)=w897, 7:T10."CRLF" ("模式（标准）"), 9:w877) -> (connection ID out=w893:refnum<k5>, data out=w880:string, error out=w863:errorcluster)
            "数据输出" <- w880
            n678 = call "数据记录.vi"("写入字段"=w880) -> ("连接的字符串"=→"读取报文显示":string)  [unwired: 10 in]
            n679 = control-ref of="数组 2"() -> (w882:refnum<vi>)
            n680 = control-ref of="数组"() -> (w881:refnum<vi>)
            n681 = call "读取数据处理 (子VI).vi"("Array输入"=w882, "data out"=w880, "reference"=w881) -> ("数组"=→"数组":string[], "系统编码ST"=→"系统编码ST":string, "数组 2"=→"数组 2":string[], "命令编码CN"=w868:string, "设备编码MN"=→"设备编码MN":string, "密码PW"=→"密码PW":string, "数据"=→"数据":string, "拆分包及应答Flag"=→"拆分包及应答Flag":string, "时间QN"=w872:string)  [unwired: 4 in]
            "命令编码CN" <- w868
            "时间QN" <- w872
            n682 = Search/Split String(string=w872, search string/char (-)="QN=" ("搜索字符串/字符(-)")) -> (match + rest of string=w870:string)  [unwired: 1 in, 2 out]
            n683 = String Subset(string=w870, offset (0)=3 ("偏移量(0)")) -> (substring=→"QN":string)  [unwired: 1 in]
            n684 = Search/Split String(string=w868, search string/char (-)="CN=" ("搜索字符串/字符(-)")) -> (match + rest of string=w861:string)  [unwired: 1 in, 2 out]
            n685 = String Subset(string=w861, offset (0)=3 ("偏移量(0)")) -> (substring=w858:string)  [unwired: 1 in]
            n686 = case shown="\"3080\", \"3081\", \"3082\", \"3083\", \"3084\", \"3085\", \"3086\"" w858 {
              tunnel: w867 -> [w900 w902 w910 w913 w916 w919 w926 w944 w961 w977 w994 w1011 w1095 w1116 w1122 w1135 w1151]
              tunnel: [w900 w902 w910 w913 w916 w919 w926 w944 w961 w977 w994 w1011 w1095 w1116 w1122 w1135 w1151] -> w865
              tunnel: [T1."读取数据" ("元素") T1."发送数据" ("元素") T1."发送数据" ("元素") T1."发送数据" ("元素") T1."发送数据" ("元素") T1."发送数据" ("元素") T1."发送数据" ("元素") T1."发送数据" ("元素") T1."发送数据" ("元素") T1."发送数据" ("元素") T1."发送数据" ("元素") T1."发送数据" ("元素") T1."发送数据" ("元素") T1."发送数据" ("元素") T1."发送数据" ("元素") T1."发送数据" ("元素") T1."发送数据" ("元素")] -> w864
              tunnel: w858 -> [_ _ _ _ _ _ _ _ _ _ _ _ _ _ _ _ w1138]
              frame "", Default {
              }
              frame "1000" {
                # "发回给平台"
                # "反控指令"
                # "3042~3086"
                # "1000"
                n687 = property on="数据" class="Str"() -> ("Value"=w908:string)  [unwired: 2 in, 2 out]
                n688 = String Subset(string=w908, offset (0)=9 ("偏移量(0)"), length (rest)=1 ("长度（剩余）")) -> (substring=w905:string)
                n689 = Decimal String To Number(string=w905) -> (number=→"设置超时时间/min":i32)  [unwired: 2 in, 1 out]
                n690 = local write "table元素"("反控命令" ("新元素/子数组")) -> ()
              }
              frame "1014" {
                # "1014"
                n691 = local write "table元素"("提取数采仪时间") -> ()
              }
              frame "1015" {
                # "设置数采仪时间"
                n692 = local write "table元素"("反控命令" ("新元素/子数组")) -> ()
              }
              frame "1061" {
                # "1061"
                n693 = local write "table元素"("提取实时数据间隔") -> ()
              }
              frame "1062" {
                # "发回给平台"
                # "反控指令"
                # "3042~3086"
                # "设置数据发送时间间隔"
                # "1062"
                n694 = property on="数据" class="Str"() -> ("Value"=w924:string)  [unwired: 2 in, 2 out]
                n695 = String Subset(string=w924, offset (0)=12 ("偏移量(0)")) -> (substring=w922:string)  [unwired: 1 in]
                n696 = Decimal String To Number(string=w922) -> (number=w921:i32)  [unwired: 2 in, 1 out]
                n697 = property on="实时数据发送时间间隔/min" class="DigNum (严格)"("Value"=w921) -> ()  [unwired: 2 in, 2 out]
                n698 = local write "table元素"("反控命令" ("新元素/子数组")) -> ()
              }
              frame "2011" {
                w931 = 0 ("数值")
                # "2011提取实时数据"
                n699 = local read "数据"() -> (w932:string)
                n700 = String Subset(string=w932, offset (0)=10 ("偏移量(0)"), length (rest)=14 ("长度（剩余）")) -> (substring=w928:string)
                n701 = String Subset(string=w932, offset (0)=33 ("偏移量(0)"), length (rest)=14 ("长度（剩余）")) -> (substring=w930:string)
                n702 = global write "全局 小时数据发送次数.vi" "小时数据发送次数"(w931) -> ()
                n703 = call "格式时间字符串.vi"("字符串"=w928) -> ("连接的字符串"=w927:string)  [unwired: 10 in]
                n704 = call "格式时间字符串.vi"("字符串"=w930) -> ("连接的字符串"=w929:string)  [unwired: 10 in]
                n705 = global write "全局1.vi" "枚举"(w931) -> ()
                n706 = global write "起始时间.vi" "结束时间"(w929) -> ()
                n707 = global write "起始时间.vi" "起始时间"(w927) -> ()
                n708 = flat-sequence {
                  frame #0 {
                    w937 = "提取实时数据" ("新元素/子数组")
                    n709 = global write "全局 实时数据参数.vi" "实时数据参数"("水样测试") -> ()
                    n710 = call "从数据库获取数据通用可配置(子VI).vi"("table输入"=w937, "列队名（唯一）"=w937) -> ()  [unwired: 8 in, 2 out]
                  }
                  frame #1 {
                    # "数据处理整合"
                    n711 = call "数据处理整合 (子VI).vi"("枚举"=enum16{"实时数据排序", "小时数据排序"}."实时数据排序") -> ("已排序的数组"=w940:string[])  [unwired: 10 in]
                    n712 = Array Size(array=w940) -> (size(s)=w941:i32)
                    n713 = global write "全局 数据数组大小.vi" "数据数组大小"(w941) -> ()
                    n714 = local write "table元素"("提取实时数据" ("新元素/子数组")) -> ()
                  }
                }
              }
              frame "2061" {
                w945 = 0 ("数值")
                n715 = flat-sequence {
                  frame #0 {
                    # "格式时间"
                    # "2061、提取小时数据"
                    n716 = local read "数据"() -> (w952:string)
                    n717 = String Subset(string=w952, offset (0)=33 ("偏移量(0)"), length (rest)=14 ("长度（剩余）")) -> (substring=w947:string)
                    n718 = String Subset(string=w952, offset (0)=10 ("偏移量(0)"), length (rest)=14 ("长度（剩余）")) -> (substring=w948:string)
                    n719 = call "格式时间字符串.vi"("字符串"=w948) -> ("连接的字符串"=w949:string)  [unwired: 10 in]
                    n720 = call "格式时间字符串.vi"("字符串"=w947) -> ("连接的字符串"=w946:string)  [unwired: 10 in]
                    n721 = global write "全局 时间.vi" "小时数据时间"(w949) -> ()
                    n722 = global write "全局 时间2.vi" "小时数据时间2"(w946) -> ()
                  }
                  frame #1 {
                    w955 = "小时数据" ("名称（未命名）")
                    # "提取COD、氨氮、多参数、总磷、总氮数据"
                    n723 = call "从数据库获取数据通用可配置(子VI).vi"("table输入"=w955, "列队名（唯一）"=w955) -> ()  [unwired: 8 in, 2 out]
                  }
                  frame #2 {
                    # "数据处理整合"
                    n724 = local write "table元素"("小时数据" ("新元素/子数组")) -> ()
                    n725 = call "数据处理整合 (子VI).vi"("枚举"=enum16{"实时数据排序", "小时数据排序"}."实时数据排序") -> ("已排序的数组"=w958:string[])  [unwired: 10 in]
                    n726 = Array Size(array=w958) -> (size(s)=w957:i32)
                    n727 = global write "全局 数据数组大小.vi" "数据数组大小"(w957) -> ()
                  }
                }
                n728 = global write "全局 小时数据发送次数.vi" "小时数据发送次数"(w945) -> ()
                n729 = global write "全局1.vi" "枚举"(w945) -> ()
              }
              frame "2062" {
                w962 = 0 ("数值")
                n730 = flat-sequence {
                  frame #0 {
                    # "格式时间"
                    # "2062、提取核查数据"
                    n731 = local read "数据"() -> (w969:string)
                    n732 = String Subset(string=w969, offset (0)=33 ("偏移量(0)"), length (rest)=14 ("长度（剩余）")) -> (substring=w964:string)
                    n733 = String Subset(string=w969, offset (0)=10 ("偏移量(0)"), length (rest)=14 ("长度（剩余）")) -> (substring=w965:string)
                    n734 = call "格式时间字符串.vi"("字符串"=w965) -> ("连接的字符串"=w966:string)  [unwired: 10 in]
                    n735 = call "格式时间字符串.vi"("字符串"=w964) -> ("连接的字符串"=w963:string)  [unwired: 10 in]
                    n736 = global write "全局 时间.vi" "时间"(w966) -> ()
                    n737 = global write "全局 时间2.vi" "时间2"(w963) -> ()
                  }
                  frame #1 {
                    w972 = "核查数据" ("新元素/子数组")
                    (unwired) "核查数据" ("名称（未命名）")
                    # "提取COD、氨氮、多参数、总磷、总氮数据"
                    n738 = call "从数据库获取数据通用可配置(子VI).vi"("table输入"=w972, "列队名（唯一）"=w972) -> ()  [unwired: 8 in, 2 out]
                  }
                  frame #2 {
                    # "数据处理整合"
                    n739 = local write "table元素"("核查数据" ("新元素/子数组")) -> ()
                    n740 = call "数据处理整合 (子VI).vi"() -> ("已排序的数组"=w973:string[])  [unwired: 11 in]
                    n741 = Array Size(array=w973) -> (size(s)=w974:i32)
                    n742 = global write "全局 数据数组大小.vi" "数据数组大小"(w974) -> ()
                  }
                }
                n743 = global write "全局 小时数据发送次数.vi" "小时数据发送次数"(w962) -> ()
                n744 = global write "全局1.vi" "枚举"(w962) -> ()
              }
              frame "2065" {
                w978 = 0 ("数值")
                n745 = flat-sequence {
                  frame #0 {
                    # "格式时间"
                    # "2065、提取零点核查数据"
                    n746 = local read "数据"() -> (w987:string)
                    n747 = global write "全局 实时数据参数.vi" "实时数据参数"("空白测试" ("新元素/子数组")) -> ()
                    n748 = local write "table元素"("实时数据" ("新元素/子数组")) -> ()
                    n749 = String Subset(string=w987, offset (0)=33 ("偏移量(0)"), length (rest)=14 ("长度（剩余）")) -> (substring=w982:string)
                    n750 = String Subset(string=w987, offset (0)=10 ("偏移量(0)"), length (rest)=14 ("长度（剩余）")) -> (substring=w983:string)
                    n751 = call "格式时间字符串.vi"("字符串"=w983) -> ("连接的字符串"=w984:string)  [unwired: 10 in]
                    n752 = call "格式时间字符串.vi"("字符串"=w982) -> ("连接的字符串"=w981:string)  [unwired: 10 in]
                    n753 = global write "全局 时间.vi" "时间"(w984) -> ()
                    n754 = global write "全局 时间2.vi" "时间2"(w981) -> ()
                  }
                  frame #1 {
                    w990 = "空白测试" ("新元素/子数组")
                    n755 = call "从数据库获取数据通用可配置(子VI).vi"("table输入"=w990, "列队名（唯一）"=w990) -> ()  [unwired: 8 in, 2 out]
                  }
                  frame #2 {
                    # "数据处理整合"
                    n756 = call "数据处理整合 (子VI).vi"() -> ("已排序的数组"=w991:string[])  [unwired: 11 in]
                    n757 = Array Size(array=w991) -> (size(s)=w992:i32)
                    n758 = global write "全局 数据数组大小.vi" "数据数组大小"(w992) -> ()
                  }
                }
                n759 = global write "全局 小时数据发送次数.vi" "小时数据发送次数"(w978) -> ()
                n760 = global write "全局1.vi" "枚举"(w978) -> ()
              }
              frame "2066" {
                w995 = 0 ("数值")
                n761 = flat-sequence {
                  frame #0 {
                    # "格式时间"
                    # "2066、提取跨度核查数据"
                    n762 = local read "数据"() -> (w1004:string)
                    n763 = String Subset(string=w1004, offset (0)=33 ("偏移量(0)"), length (rest)=14 ("长度（剩余）")) -> (substring=w999:string)
                    n764 = String Subset(string=w1004, offset (0)=10 ("偏移量(0)"), length (rest)=14 ("长度（剩余）")) -> (substring=w1000:string)
                    n765 = global write "全局 实时数据参数.vi" "实时数据参数"("跨度核查" ("新元素/子数组")) -> ()
                    n766 = local write "table元素"("实时数据" ("新元素/子数组")) -> ()
                    n767 = call "格式时间字符串.vi"("字符串"=w1000) -> ("连接的字符串"=w1001:string)  [unwired: 10 in]
                    n768 = call "格式时间字符串.vi"("字符串"=w999) -> ("连接的字符串"=w998:string)  [unwired: 10 in]
                    n769 = global write "全局 时间.vi" "时间"(w1001) -> ()
                    n770 = global write "全局 时间2.vi" "时间2"(w998) -> ()
                  }
                  frame #1 {
                    w1007 = "跨度核查" ("新元素/子数组")
                    (unwired) "跨度核查" ("名称（未命名）")
                    # "提取COD、氨氮、多参数、总磷、总氮数据"
                    n771 = call "从数据库获取数据通用可配置(子VI).vi"("table输入"=w1007, "列队名（唯一）"=w1007) -> ()  [unwired: 8 in, 2 out]
                  }
                  frame #2 {
                    # "数据处理整合"
                    n772 = call "数据处理整合 (子VI).vi"() -> ("已排序的数组"=w1009:string[])  [unwired: 11 in]
                    n773 = Array Size(array=w1009) -> (size(s)=w1008:i32)
                    n774 = global write "全局 数据数组大小.vi" "数据数组大小"(w1008) -> ()
                  }
                }
                n775 = global write "全局 小时数据发送次数.vi" "小时数据发送次数"(w995) -> ()
                n776 = global write "全局1.vi" "枚举"(w995) -> ()
              }
              frame "3020" {
                n777 = flat-sequence {
                  frame #0 {
                    w1012 = 0 ("数值")
                    # "3020、提取日志"
                    # "格式时间"
                    n778 = local read "数据"() -> (w1014:string)
                    n779 = Search/Split String(string=w1014, search string/char (-)="BeginTime=" ("搜索字符串")) -> (match + rest of string=w1013:string)  [unwired: 1 in, 2 out]
                    n780 = String Subset(string=w1013, offset (0)=10 ("偏移量(0)"), length (rest)=14 ("长度（剩余）")) -> (substring=w1018:string)
                    n781 = String Subset(string=w1013, offset (0)=33 ("偏移量(0)"), length (rest)=14 ("长度（剩余）")) -> (substring=w1017:string)
                    n782 = call "格式时间字符串.vi"("字符串"=w1018) -> ("连接的字符串"=w1019:string)  [unwired: 10 in]
                    n783 = call "格式时间字符串.vi"("字符串"=w1017) -> ("连接的字符串"=w1016:string)  [unwired: 10 in]
                    n784 = global write "全局 时间2.vi" "时间2"(w1016) -> ()
                    n785 = global write "全局 时间.vi" "时间"(w1019) -> ()
                    n786 = global write "全局 小时数据发送次数.vi" "小时数据发送次数"(w1012) -> ()
                    n787 = global write "全局1.vi" "枚举"(w1012) -> ()
                  }
                  frame #1 {
                    # "按需求提取COD、氨氮、总磷、总氮日志"
                    # "按需求提取COD、氨氮、总磷、总氮日志"
                    n788 = control-ref of="数据"() -> (w1026:refnum<vi>)
                    n789 = call "日志报警参数选择 (子VI).vi"("String输入"=w1026) -> ("输出簇"=w1027:T11)  [unwired: 9 in, 1 out]
                    n790 = Obtain Queue(name (unnamed)="操作日志报警信息" ("名称（未命名）"), element data type=enum16{"CODMn", "氨氮", "总磷", "总氮", "数采仪"}."CODMn") -> (queue out=w1025:refnum<queue>, error out=w1039:errorcluster)  [unwired: 3 in, 1 out]
                    n791 = Unbundle By Name(w1027) -> ("高锰酸盐"=w1028:string, "氨氮"=w1029:string, "总磷"=w1030:string, "总氮"=w1031:string, "数采仪"=w1032:string, "高锰酸盐"=w1033:bool, "氨氮"=w1034:bool, "总磷"=w1035:bool, "总氮"=w1036:bool, "数采仪"=w1037:bool)
                    n792 = Build Array(w1028, w1029, w1030, w1031, w1032) -> (w1024:string[])
                    n793 = Build Array(w1033, w1034, w1035, w1036, w1037) -> (w1038:bool[])
                    n794 = for {
                      tunnel: w1038 -> [w1043] mode=indexing
                      tunnel: w1025 -> [w1042]
                      i -> [w1044]
                      n795 = case shown="真" w1043 {
                        tunnel: w1044 -> [_ w1046]
                        tunnel: w1042 -> [_ w1045]
                        frame False {
                        }
                        frame True {
                          n796 = call "提取日志报警参数入列队 (子VI).vi"("枚举"=w1046, "队列输入"=w1045) -> ()  [unwired: 10 in]
                        }
                      }
                    }
                    n797 = while {
                      shift-right: [w1059] -> _
                      shift-left: w1025 -> [w1060]
                      tunnel: w1039 -> [w1058]
                      tunnel: w1024 -> [w1053]
                      stop <- w1055 stop-if-true
                      n798 = Dequeue Element(queue=w1060, error in (no error)=w1058) -> (queue out=w1057:refnum<queue>, element=w1052:enum16{"CODMn", "氨氮", "总磷", "总氮", "数采仪"})  [unwired: 1 in, 2 out]
                      n799 = Index Array(array=w1053) -> (element #1=w1051:string, element #2=w1050:string, element #3=w1049:string, element #4=w1048:string, element #5=w1047:string)  [unwired: 5 in]
                      n800 = case shown="\"CODMn\"" w1052 {
                        tunnel: w1057 -> [w1064 w1068 w1072 w1075 w1080]
                        tunnel: [w1064 w1068 w1072 w1075 w1080] -> w1059
                        tunnel: w1051 -> [w1061 _ _ _ _]
                        tunnel: w1050 -> [_ w1065 _ _ _]
                        tunnel: w1049 -> [_ _ w1069 _ _]
                        tunnel: w1048 -> [_ _ _ w1073 _]
                        tunnel: w1047 -> [_ _ _ _ w1077]
                        frame "CODMn" {
                          n801 = call "数据表比对.vi"("仪器日志参数"="CODMn" ("元素"), "table输入"=w1061) -> ("待发送数据"=w1062:string[][])  [unwired: 6 in, 3 out]
                          n802 = global write "全局 所有参数.vi" "CODMn"(w1062) -> ()
                        }
                        frame "氨氮" {
                          n803 = call "数据表比对.vi"("仪器日志参数"="氨氮" ("元素"), "table输入"=w1065) -> ("待发送数据"=w1066:string[][])  [unwired: 6 in, 3 out]
                          n804 = global write "全局 所有参数.vi" "氨氮"(w1066) -> ()
                        }
                        frame "总磷" {
                          n805 = call "数据表比对.vi"("仪器日志参数"="总磷" ("元素"), "table输入"=w1069) -> ("待发送数据"=w1070:string[][])  [unwired: 6 in, 3 out]
                          n806 = global write "全局 所有参数.vi" "总磷"(w1070) -> ()
                        }
                        frame "总氮" {
                          n807 = call "数据表比对.vi"("仪器日志参数"="总氮" ("元素"), "table输入"=w1073) -> ("待发送数据"=w1074:string[][])  [unwired: 6 in, 3 out]
                          n808 = global write "全局 所有参数.vi" "总氮"(w1074) -> ()
                        }
                        frame "数采仪" {
                          n809 = call "数据表比对.vi"("仪器日志参数"="系统" ("元素"), "table输入"=w1077) -> ("待发送数据"=w1078:string[][])  [unwired: 6 in, 3 out]
                          n810 = global write "全局 所有参数.vi" "DO"(w1078) -> ()
                        }
                      }
                      n811 = Get Queue Status(queue=w1057) -> (# elements in queue=w1056:i32)  [unwired: 2 in, 7 out]
                      n812 = Wait (ms)(milliseconds to wait=u32 300 ("等待时间（毫秒）")) -> ()  [unwired: 1 out]
                      n813 = Equal To 0?(x=w1056) -> (x = 0?=w1055:bool)
                    }
                  }
                  frame #2 {
                    # "数据处理整合"
                    n814 = local read "数据"() -> (w1088:string)
                    n815 = call "数据处理整合 (子VI).vi"("枚举"=enum16{"实时数据排序", "小时数据排序"}."实时数据排序") -> ("已排序的数组"=w1089:string[])  [unwired: 10 in]
                    n816 = Search/Split String(string=w1088, search string/char (-)="InfoId=" ("搜索字符串/字符(-)")) -> (match + rest of string=w1086:string)  [unwired: 1 in, 2 out]
                    n817 = Array Size(array=w1089) -> (size(s)=w1090:i32)
                    n818 = String Subset(string=w1086, offset (0)=7 ("偏移量(0)"), length (rest)=6 ("长度（剩余）")) -> (substring=w1083:string)
                    n819 = case shown="\"i11001\", \"i21001\"" w1083 {
                      tunnel: ["报警信息" ("新元素/子数组") "操作日志" ("新元素/子数组")] -> w1082
                      frame "i12001", Default {
                      }
                      frame "i11001", "i21001" {
                      }
                    }
                    n820 = global write "全局 数据数组大小.vi" "数据数组大小"(w1090) -> ()
                    n821 = local write "table元素"(w1082) -> ()
                  }
                }
              }
              frame "3042" {
                # "发命令给中控"
                # "反控指令"
                # "0维护，1常规，2应急，3质控"
                # "反控指令\n切换运行模式"
                n822 = local write "table元素"("反控命令" ("新元素/子数组")) -> ()
                n823 = property on="数据" class="Str"() -> ("Value"=w1107:string)  [unwired: 2 in, 2 out]
                n824 = Search/Split String(string=w1107, search string/char (-)="RunMode" ("搜索字符串/字符(-)")) -> (match + rest of string=w1105:string)  [unwired: 1 in, 2 out]
                n825 = String Subset(string=w1105, offset (0)=8 ("偏移量(0)"), length (rest)=1 ("长度（剩余）")) -> (substring=w1102:string)
                n826 = case shown="\"1\"" w1102 {
                  tunnel: [u16 0 ("新元素/子数组") u16 1 ("新元素/子数组") u16 2 ("新元素/子数组") u16 3 ("新元素/子数组")] -> w1096
                  frame "0", Default {
                  }
                  frame "1" {
                  }
                  frame "2" {
                  }
                  frame "3" {
                  }
                }
                n827 = Insert Into Array(array=u16[] [] ("holding register values"), index=0 ("索引"), new element=w1096) -> (w1097:u16[])
                n828 = call "Modbus Master.vi"("Unit ID"=u8 1, "holding register values"=w1097, "starting address"=u16 0) -> ()  [unwired: 8 in, 1 out]
              }
              frame "3044" {
                # "发命令给中控"
                # "发回给平台"
                # "反控指令"
                # "3042~3086"
                # "反控指令\n单次测量"
                # "3044"
                n829 = local write "table元素"("反控命令" ("新元素/子数组")) -> ()
                n830 = call "Modbus Master.vi"("Unit ID"=u8 1, "holding register values"=u16[] [1], "starting address"=u16 2) -> ()  [unwired: 8 in, 1 out]
              }
              frame "3045" {
                # "发命令给中控"
                # "发回给平台"
                # "反控指令"
                # "3042~3086"
                # "反控指令\n急停"
                # "3045"
                n831 = local write "table元素"("反控命令" ("新元素/子数组")) -> ()
                n832 = call "Modbus Master.vi"("Unit ID"=u8 1, "holding register values"=u16[] [1], "starting address"=u16 3) -> ()  [unwired: 8 in, 1 out]
              }
              frame "3056" {
                # "设置测量时间间隔"
                # "发命令给中控"
                # "发回给平台"
                n833 = property on="数据" class="Str"() -> ("Value"=w1129:string)  [unwired: 2 in, 2 out]
                n834 = Search/Split String(string=w1129, search string/char (-)="RunInterval" ("搜索字符串/字符(-)")) -> (match + rest of string=w1130:string)  [unwired: 1 in, 2 out]
                n835 = Decimal String To Number(string=w1130, offset=12 ("偏移量(0)")) -> (number=w1125:i32)  [unwired: 1 in, 1 out]
                n836 = Insert Into Array(array=u16[] [] ("holding register values"), index=0 ("索引"), new element=w1125) -> (w1124:u16[])
                n837 = local write "table元素"("反控命令" ("新元素/子数组")) -> ()
                n838 = call "Modbus Master.vi"("Unit ID"=u8 1, "holding register values"=w1124, "starting address"=u16 14) -> ()  [unwired: 8 in, 1 out]
              }
              frame "3080", "3081", "3082", "3083", "3084", "3085", "3086" {
                # "30 启动标液核查  1CODmn  2 氨氮  3总磷  4总氮  5CODCr\n31 加标回收\n32 平行样测试\n33 零点核查\n34 跨度核查\n35 校零\n36 校标"
                # "1CODmn  2 氨氮  3总磷  4总氮  5CODCr"
                # "启动单台仪器标液核查"
                # "发命令给中控"
                # "发回给平台"
                n839 = property on="数据" class="Str"() -> ("Value"=w1148:string)  [unwired: 2 in, 2 out]
                n840 = Search/Split String(string=w1148, search string/char (-)="PolId" ("搜索字符串/字符(-)")) -> (match + rest of string=w1143:string)  [unwired: 1 in, 2 out]
                n841 = String Subset(string=w1143, offset (0)=6 ("偏移量(0)"), length (rest)=6 ("长度（剩余）")) -> (substring=w1140:string)
                n842 = case shown="\"w01019\"" w1140 {
                  tunnel: [0 ("长度（剩余）") 1 ("长度（剩余）") 2 ("长度（剩余）") 3 ("长度（剩余）") 4 ("长度（剩余）") 5 ("长度（剩余）")] -> w1139
                  frame "", Default {
                  }
                  frame "w01019" {
                  }
                  frame "w21003" {
                  }
                  frame "w21011" {
                  }
                  frame "w21001" {
                  }
                  frame "w01018" {
                  }
                }
                n843 = Insert Into Array(array=u16[] [] ("holding register values"), index=0 ("索引"), new element=w1139) -> (w1144:u16[])
                n844 = case shown="\"3086\"" w1138 {
                  tunnel: [u16 99 ("starting address") u16 30 ("starting address") u16 31 ("starting address") u16 32 ("starting address") u16 33 ("starting address") u16 34 ("starting address") u16 35 ("starting address") u16 36 ("starting address")] -> w1137
                  frame "", Default {
                  }
                  frame "3080" {
                  }
                  frame "3081" {
                  }
                  frame "3082" {
                  }
                  frame "3083" {
                  }
                  frame "3084" {
                  }
                  frame "3085" {
                  }
                  frame "3086" {
                  }
                }
                n845 = local write "table元素"("反控命令" ("新元素/子数组")) -> ()
                n846 = call "Modbus Master.vi"("Unit ID"=u8 1, "holding register values"=w1144, "starting address"=w1137) -> ()  [unwired: 8 in, 1 out]
              }
            }
            n847 = Enqueue Element(queue=w865, element=w864, timeout in ms (-1)=1000 ("超时毫秒(-1)")) -> ()  [unwired: 1 in, 3 out]
          }
          frame "发送数据" {
            # "table输入，选择命令编码、发送哪些数据"
            n848 = local read "table元素"() -> (w1171:string)
            n849 = case shown="\"反控命令\"" w1171 {
              tunnel: w1170 -> [w1185 w1189 w1194]
              tunnel: [w1183 w1188 w1192] -> w1168
              tunnel: [w1184 w1187 w1193] -> w1169
              frame "", Default {
                n850 = Increment(x=w1185) -> (x+1=w1184:i32)
                n851 = global write "全局1.vi" "枚举"(w1185) -> ()
                n852 = Greater Or Equal?(x=w1184, y=3) -> (x >= y?=w1183:bool)
              }
              frame "反控命令" {
                n853 = Increment(x=w1189) -> (x+1=w1187:i32)
                n854 = global write "全局 反控命令枚举.vi" "反控命令枚举"(w1189) -> ()
                n855 = Greater Or Equal?(x=w1187, y=2) -> (x >= y?=w1188:bool)
              }
              frame "报警信息", "操作日志", "核查数据", "跨度核查", "零点核查", "实时数据", "提取实时数据", "小时数据" {
                n856 = global read "全局 小时数据发送次数.vi" "小时数据发送次数"() -> (w1196:i32)
                n857 = global read "全局 数据数组大小.vi" "数据数组大小"() -> (w1191:i32)
                n858 = Greater Or Equal?(x=w1196, y=w1191) -> (x >= y?=w1197:bool)
                n859 = case shown="真" w1197 {
                  tunnel: w1194 -> [w1202 w1209]
                  tunnel: [w1202 w1203] -> w1198
                  frame False {
                  }
                  frame True {
                    n860 = global read "全局 小时数据发送次数.vi" "小时数据发送次数"() -> (w1208:i32)
                    n861 = global read "全局 数据数组大小.vi" "数据数组大小"() -> (w1205:i32)
                    n862 = Equal To 0?(x=w1205) -> (x = 0?=w1206:bool)
                    n863 = Equal To 0?(x=w1208) -> (x = 0?=w1207:bool)
                    n864 = And(x=w1207, y=w1206) -> (x .and. y?=w1204:bool)
                    n865 = case shown="假" w1204 {
                      tunnel: w1209 -> [w1211 _]
                      tunnel: [w1210 0 ("索引")] -> w1203
                      frame False {
                        n866 = Increment(x=w1211) -> (x+1=w1210:i32)
                      }
                      frame True {
                      }
                    }
                  }
                }
                n867 = Equal To 0?(x=w1198) -> (x = 0?=w1199:bool)
                n868 = global write "全局1.vi" "枚举"(w1198) -> ()
                n869 = case shown="真" w1199 {
                  tunnel: w1198 -> [w1200 _]
                  tunnel: [w1200 1] -> w1193
                  frame False {
                  }
                  frame True {
                  }
                }
                n870 = Greater Or Equal?(x=w1193, y=2) -> (x >= y?=w1192:bool)
              }
            }
            n871 = case shown="假" w1168 {
              tunnel: w1169 -> [w1213 _]
              tunnel: [w1213 1 ("索引")] -> w1173
              frame False {
              }
              frame True {
              }
            }
            n872 = flat-sequence {
              tunnel: w1182 -> [w1217]
              tunnel: "table元素" -> [w1223]
              tunnel: w1178 -> [w1222]
              tunnel: [w1225] -> w1177
              tunnel: [w1218] -> w1176
              tunnel: [w1228] -> w1174
              tunnel: [w1229] -> w1179
              tunnel: w1177 -> [w1229]
              tunnel: w1176 -> [w1228]
              tunnel: w1175 -> [w1227]
              tunnel: w1168 -> [w1226]
              frame #0 {
                # "数据记录"
                # "数据编码"
                n873 = local read "QN"() -> (w1215:string)
                n874 = call "数据编码.vi"("table输入"=w1223, "错误常量 2"=w1222, "QN"=w1215, "MN"="MN", "PW"="PW") -> ("错误常量"=w1221:errorcluster, "通讯包字符串"=w1216:string)  [unwired: 9 in]
                n875 = call "数据记录.vi"("写入字段"=w1216) -> ("连接的字符串"=→"发送报文显示":string)  [unwired: 10 in]
                n876 = TCP Write(connection ID=w1217, data in=w1216, error in (no error)=w1221) -> (connection ID out=w1225:refnum<k5>, error out=w1218:errorcluster)  [unwired: 1 in, 1 out]
              }
              frame #1 {
                n877 = case shown="真" w1226 {
                  tunnel: w1227 -> [w1230 w1242]
                  frame False {
                    n878 = Enqueue Element(queue=w1230, element=T1."发送数据" ("元素")) -> ()  [unwired: 2 in, 3 out]
                  }
                  frame True {
                    n879 = local read "TCP服务端掉线计数"() -> (w1237:i32)
                    n880 = Obtain Queue(name (unnamed)="重发掉线数据" ("名称（未命名）"), element data type=T9."水样测试") -> (queue out=w1235:refnum<queue>, error out=w1236:errorcluster)  [unwired: 3 in, 1 out]
                    n881 = Get Queue Status(queue=w1235, error in (no error)=w1236) -> (# elements in queue=w1239:i32)  [unwired: 1 in, 7 out]
                    n882 = Not Equal To 0?(x=w1239) -> (x != 0?=w1240:bool)
                    n883 = Greater Or Equal?(x=w1237, y=1) -> (x >= y?=w1241:bool)
                    n884 = And(x=w1240, y=w1241) -> (x .and. y?=w1233:bool)
                    n885 = case shown="真" w1233 {
                      tunnel: [T1."读取数据" ("元素") T1."表格比对" ("元素")] -> w1243
                      frame False {
                      }
                      frame True {
                      }
                    }
                    n886 = Enqueue Element(queue=w1242, element=w1243) -> ()  [unwired: 2 in, 3 out]
                  }
                }
              }
            }
            "数据正在发送" <- TRUE
          }
          frame "数据处理" {
            n887 = local write "try"(0.0 ("try")) -> ()
            n888 = local write "空闲时间"(0.0 ("空闲时间")) -> ()
            n889 = local read "心跳包"() -> (w1254:bool)
            n890 = Equal?(x=w1252, y="实时数据") -> (x = y?=w1250:bool)
            n891 = case shown="假" w1254 {
              tunnel: w1259 -> [w1263 _]
              tunnel: w1252 -> [w1262 _]
              frame False {
                n892 = call "插入单条数据.vi"("table输入"=w1262, "插入数据"=w1263) -> ()  [unwired: 8 in, 2 out]
              }
              frame True {
              }
            }
            n893 = Select(t=0, s=w1250, f=w1248) -> (s? t:f=w1249:i32)
            n894 = Enqueue Element(queue=w1258, element=T1."表格比对" ("元素"), timeout in ms (-1)=1000 ("超时毫秒(-1)")) -> ()  [unwired: 1 in, 3 out]
          }
        }
      }
      frame Error {
        n895 = Unbundle By Name(w1267) -> ("code"=w1266:i32)
        n896 = case shown="63" w1266 {
          tunnel: w1273 -> [w1279 w1297 w1330 w1345]
          tunnel: w1267 -> [w1277 w1298 w1331 w1344]
          tunnel: [w1278 w1290 w1323 w1345] -> w1272
          tunnel: [w1275 w1296 w1329 w1344] -> w1271
          tunnel: w1265 -> [w1280 w1291 w1324 w1341]
          frame 0, Default {
            n897 = Flush Queue(queue=w1280) -> (queue out=w1274:refnum<queue>)  [unwired: 1 in, 2 out]
            n898 = Enqueue Element(queue=w1274, element=T1."初始化" ("元素"), timeout in ms (-1)=1000 ("超时毫秒(-1)")) -> ()  [unwired: 1 in, 3 out]
            n899 = TCP Close Connection(connection ID=w1279, error in (no error)=w1277) -> (connection ID out=w1278:refnum<k5>, error out=w1276:errorcluster)  [unwired: 1 in]
            n900 = call <vilib>:"Clear Errors.vi"("error in (no error)"=w1276) -> ("error out"=w1275:errorcluster)  [unwired: 5 in, 1 out]
          }
          frame 63 {
            # "TCP服务器端口掉线"
            n901 = local read "数据正在发送"() -> (w1287:bool)
            "数据接收中断" <- w1287
            n902 = Flush Queue(queue=w1291) -> (queue out=w1292:refnum<queue>)  [unwired: 1 in, 2 out]
            n903 = property on="TCP服务端掉线计数" class="DigNum (严格)"() -> ("Value"=w1286:i32)  [unwired: 2 in, 2 out]
            n904 = call <vilib>:"Boolean Crossing PtByPt.vi"("direction"=enum16{"either", "false-true", "true-false"}."false-true", "input"=w1287) -> ("crossing"=w1288:bool)  [unwired: 1 in]
            n905 = Less Or Equal?(x=w1286, y=1) -> (x <= y?=w1284:bool)
            n906 = Enqueue Element(queue=w1292, element=T1."初始化" ("元素"), timeout in ms (-1)=1000 ("超时毫秒(-1)")) -> ()  [unwired: 1 in, 3 out]
            n907 = case shown="真" w1288 {
              frame False {
              }
              frame True {
                # "判定数据为空时不写入临时表格"
                n908 = call "每个元素都写入临时表格 (子VI).vi"("组合框"="小时数据存储") -> ()  [unwired: 10 in, 1 out]
              }
            }
            n909 = case shown="真" w1284 {
              frame False {
                n910 = global write "全局 数据发送重叠.vi" "TCP掉线时间节点"("TCP掉线时间节点") -> ()
                n911 = local write "TCP掉线时间节点"("TCP掉线时间节点") -> ()
              }
              frame True {
                n912 = Get Date/Time In Seconds() -> (seconds since 1Jan1904=w1312:timestamp)
                n913 = Format Date/Time String(time format string (%c)="%Y%m%d%H%M%S%3u" ("时间格式字符串(%c)"), seconds (now)=w1312) -> (date/time string=w1314:string)  [unwired: 1 in]
                n914 = call "格式时间字符串.vi"("字符串"=w1314) -> ("连接的字符串"=w1302:string)  [unwired: 10 in]
                n915 = local write "TCP掉线时间节点"(w1302) -> ()
                n916 = call <vilib>:"Application Directory.vi"() -> ("Application Directory"=w1310:path)
                n917 = Build Path(base path=w1310, name or relative path="data\\Set.ini" ("名称或相对路径")) -> (appended path=w1311:path)
                n918 = call <vilib>:"Open Config Data.vi"("configuration file path"=w1311) -> ("error out"=w1307:errorcluster, "refnum"=w1308:T6)  [unwired: 8 in, 1 out]
                n919 = call-poly <vilib>:"Write Key.vi"("section"="掉线时间存储", "error in (no error)"=w1307, "value"=w1302, "key"="掉线时间", "refnum"=w1308) -> ("error out"=w1305:errorcluster, "refnum out"=w1306:T6)  [unwired: 4 in, 1 out]
                n920 = call <vilib>:"Close Config Data.vi"("error in (no error)"=w1305, "refnum"=w1306) -> ()  [unwired: 8 in, 2 out]
              }
            }
            n921 = property on="TCP服务端掉线计数" class="DigNum (严格)"() -> ("Value"=w1295:i32)  [unwired: 2 in, 2 out]
            n922 = TCP Close Connection(connection ID=w1297, error in (no error)=w1298) -> (connection ID out=w1290:refnum<k5>, error out=w1299:errorcluster)  [unwired: 1 in]
            n923 = Increment(x=w1295) -> (x+1=w1293:i32)
            n924 = property on="TCP服务端掉线计数" class="DigNum (严格)"("Value"=w1293) -> ()  [unwired: 2 in, 2 out]
            n925 = call <vilib>:"Clear Errors.vi"("error in (no error)"=w1299) -> ("error out"=w1296:errorcluster)  [unwired: 5 in, 1 out]
            n926 = global write "全局 数据发送重叠.vi" "掉线指示灯"(TRUE ("掉线指示灯")) -> ()
          }
          frame 54 {
            # "TCP服务器端口掉线"
            n927 = local read "数据正在发送"() -> (w1320:bool)
            "数据接收中断 2" <- w1320
            n928 = Flush Queue(queue=w1324) -> (queue out=w1325:refnum<queue>)  [unwired: 1 in, 2 out]
            n929 = property on="TCP服务端掉线计数" class="DigNum (严格)"() -> ("Value"=w1319:i32)  [unwired: 2 in, 2 out]
            n930 = call <vilib>:"Boolean Crossing PtByPt.vi"("direction"=enum16{"either", "false-true", "true-false"}."false-true", "input"=w1320) -> ("crossing"=w1321:bool)  [unwired: 1 in]
            n931 = Less Or Equal?(x=w1319, y=1) -> (x <= y?=w1317:bool)
            n932 = Enqueue Element(queue=w1325, element=T1."初始化" ("元素"), timeout in ms (-1)=1000 ("超时毫秒(-1)")) -> ()  [unwired: 1 in, 3 out]
            n933 = case shown="真" w1321 {
              frame False {
              }
              frame True {
                # "判定数据为空时不写入临时表格"
                n934 = call "每个元素都写入临时表格 (子VI).vi"("组合框"="小时数据存储") -> ()  [unwired: 10 in, 1 out]
              }
            }
            n935 = case shown="假" w1317 {
              frame False {
                n936 = local read "TCP掉线时间节点"() -> (w1334:string)
                n937 = global write "全局 数据发送重叠.vi" "TCP掉线时间节点"(w1334) -> ()
                n938 = local write "TCP掉线时间节点"(w1334) -> ()
              }
              frame True {
                n939 = Get Date/Time In Seconds() -> (seconds since 1Jan1904=w1336:timestamp)
                n940 = Format Date/Time String(time format string (%c)="%Y%m%d%H%M%S%3u" ("时间格式字符串(%c)"), seconds (now)=w1336) -> (date/time string=w1338:string)  [unwired: 1 in]
                n941 = call "格式时间字符串.vi"("字符串"=w1338) -> ("连接的字符串"=w1335:string)  [unwired: 10 in]
                n942 = local write "TCP掉线时间节点"(w1335) -> ()
              }
            }
            n943 = property on="TCP服务端掉线计数" class="DigNum (严格)"() -> ("Value"=w1328:i32)  [unwired: 2 in, 2 out]
            n944 = TCP Close Connection(connection ID=w1330, error in (no error)=w1331) -> (connection ID out=w1323:refnum<k5>, error out=w1332:errorcluster)  [unwired: 1 in]
            n945 = Increment(x=w1328) -> (x+1=w1326:i32)
            n946 = property on="TCP服务端掉线计数" class="DigNum (严格)"("Value"=w1326) -> ()  [unwired: 2 in, 2 out]
            n947 = call <vilib>:"Clear Errors.vi"("error in (no error)"=w1332) -> ("error out"=w1329:errorcluster)  [unwired: 5 in, 1 out]
            n948 = global write "全局 数据发送重叠.vi" "掉线指示灯"(TRUE ("掉线指示灯")) -> ()
          }
          frame 56 {
            n949 = Flush Queue(queue=w1341) -> (queue out=w1342:refnum<queue>)  [unwired: 1 in, 2 out]
            n950 = Enqueue Element(queue=w1342, element=T1."读取数据" ("元素"), timeout in ms (-1)=1000 ("超时毫秒(-1)")) -> ()  [unwired: 1 in, 3 out]
          }
        }
        n951 = call <vilib>:"Clear Errors.vi"("error in (no error)"=w1271) -> ("error out"=w1270:errorcluster)  [unwired: 5 in, 1 out]
      }
    }
    "运行时间次数" <- w655
  }
  n952 = register-events(error in=w16, w17) -> (reference out=w6:refnum<event-registration>, error out=w5:errorcluster)  [unwired: 1 in]
  n953 = while {
    shift-right: [w1349] -> w9
    shift-left: w5 -> [w1348]
    shift-right: [w1350] -> w12
    shift-left: w7 -> [w1351]
    shift-right: [w1347] -> w11
    shift-left: w6 -> [w1352]
    tunnel: [w1346] -> _
    stop <- w1346 stop-if-true
    n954 = case shown="无错误" w1348 {
      selector: w1348 -> [w1354 w1388]
      tunnel: w1352 -> [w1359 w1383]
      tunnel: w1351 -> [w1358 w1384]
      tunnel: [w1357 w1384] -> w1350
      tunnel: [w1356 w1386] -> w1349
      tunnel: [w1355 FALSE ("Discard?")] -> w1346
      tunnel: [w1353 w1383] -> w1347
      frame No Error {
        n955 = event shown="[2] 前面板关闭？" {
          selector: w1359 -> [_ _ _]
          dyn-events: [_ _ _] -> w1353
          timeout: _ -> [_ _ _]
          tunnel: w1354 -> [w1362 w1372 w1381]
          tunnel: [w1362 w1372 w1380] -> w1356
          tunnel: [w1361 TRUE FALSE ("Discard?")] -> w1355
          tunnel: w1358 -> [w1360 w1370 w1382]
          tunnel: [w1360 w1370 w1379] -> w1357
          event User Event {
            # "5."
            n956 = event-data() -> ("ItemTag"=w1363:string)  [unwired: 1 in]
            n957 = case shown="\"EXIT线程二\"" w1363 {
              tunnel: [FALSE TRUE] -> w1361
              frame Default {
                n958 = Current VI's Path() -> (path=w1364:path)
                n959 = Open VI Reference(vi path=w1364) -> (vi reference=w1365:refnum<vi>)  [unwired: 5 in, 1 out]
                n960 = invoke class="VI" method="FP.Open"(reference=w1365, "Activate"=TRUE ("激活？")) -> ()  [unwired: 3 in, 5 out]
              }
              frame "EXIT线程二" {
              }
            }
          }
          event "停止 2": Value Change {
            # "5."
            n961 = event-data() -> ()  [unwired: 1 in, 2 out]
            n962 = Stop(stop? (T)=TRUE ("可见")) -> ()
          }
          event Panel Close? {
            # "4."
            n963 = event-data() -> ("VIRef"=w1375:refnum<vi>)  [unwired: 1 in, 3 out]
            n964 = invoke class="VI" method="FP.Open"(reference=w1375, "State"=T8."Hidden" ("状态")) -> ()  [unwired: 3 in, 5 out]
            n965 = call <vilib>:"ShowBalloonTip.vi"("Balloon Icon"=BalloonIcon."Information", "error in"=w1381, "Text"="欢迎使用平台发送系统", "NotifyIcon in"=w1382) -> ("error out"=w1380:errorcluster, "NotifyIcon out"=w1379:refnum<class "NotifyIcon.lvclass">)  [unwired: 6 in]
            n966 = event-data("Discard?"=TRUE ("放弃？")) -> ()  [unwired: 1 in, 1 out]
          }
        }
      }
      frame Error {
        n967 = call <vilib>:"Simple Error Handler.vi"("error in (no error)"=w1388) -> ("error out"=w1387:errorcluster)  [unwired: 4 in, 4 out]
        n968 = call <vilib>:"Clear Errors.vi"("error in (no error)"=w1387) -> ("error out"=w1386:errorcluster)  [unwired: 5 in, 1 out]
      }
    }
  }
  n969 = Unregister For Events(event registration refnum=w11, error in=w9) -> (error out=w8:errorcluster)
  n970 = call <vilib>:"Destructor.vi"("error in"=w8, "NotifyIcon"=w12) -> ("error out"=w13:errorcluster)  [unwired: 9 in]
  n971 = disable-structure shown="禁用" {
    disable-tunnel: w13 -> [w1390 _]
    frame Disabled {
      n972 = property class="App"() -> ("App.Kind"=w1389:T7)  [unwired: 2 in, 2 out]
      n973 = case shown="\"Development System\"" w1389 {
        tunnel: w1390 -> [_ _ _ _ _ _ _]
        frame "invalid app kind", Default {
        }
        frame "Development System" {
          n974 = Stop(stop? (T)=TRUE ("可见")) -> ()
        }
        frame "Run Time System" {
          n975 = Quit LabVIEW(quit? (T)=TRUE ("退出？(T)")) -> ()
        }
        frame "Student Edition" {
        }
        frame "Embedded LabVIEW" {
        }
        frame "Evaluation" {
        }
        frame "Custom" {
        }
      }
    }
    frame Enabled {
    }
  }
  n976 = call <vilib>:"Simple Error Handler.vi"("error in (no error)"=w13) -> ("error out"=→"error out":errorcluster)  [unwired: 4 in, 4 out]
  n977 = disable-structure shown="禁用" {
    frame Disabled {
      n978 = control-ref of="TCP掉线时间节点"() -> (w1393:refnum<vi>)
      n979 = global read "全局 时间2.vi" "时间2"() -> (w1396:string)
      n980 = call "读取临时表格数据 (子VI).vi"("time 2"=w1396, "表格选择"="database1.mdb", "组合框"="小时数据读取", "String输入"=w1393) -> ()  [unwired: 8 in]
    }
    frame Enabled {
    }
  }
